vi "WS1050 16 DUT Reliability HD_Cycling Ver1.8.vi"() -> ()   [LabVIEW 2012]
uses:
  WS_VCAP Driver 024/Source/WSVCAP Shell/Type Defs/WSVCAP SHL I2C DUT Mask Mode Enum.ctl
  <vilib>/Utility/file.llb/Read From Spreadsheet File (DBL).vi
panel:
  out "VISA resource name out":refnum<visa-resource-name>="GPIB0::3::INSTR"
  out "error out 2":errorcluster={"status"=TRUE, "code"=-63192, "source"="niLvFpga_Open_PXI-7813R.vi"}
  in  "Reg1_Bit Cntrl":string[](array[string])=["01", "02", "04", "08", "10", "20", "40", "80", "03", "06", "0C", "D8", "33", "66", "CC", "07", "0E", "1C", "38", "70", "E0", "0F", "1E", "3C", "78", "F0", "1F", "3E", "7C", "F8", "3F", "7E", "FC", "7F", "FE", "FD", "FB", "F7", "EF", "DF", "BF", "7F", "FC", "F9", "F3", "E7", "CF", "9F", "3F", "F8", "F1", "E3", "C7", "8F", "1F", "F0", "E1", "C3", "87", "0F", "E0", "C1", "83", "07", "C0", "81", "03", "AA", "55", "00"]
  out "date string":string="5/19/2014"
  out "PS1 Out":refnum<visa-resource-name>
  out "Ke2000 Out":refnum<visa-resource-name>="GPIB0::9::INSTR"
  in  "Tab Control":T1(tab)
  in  "No of Cmd":i64=3
  in  "Serial Number":string[][](table)=[["DUT", "SN"], ["DUT1", "1"], ["DUT2", "2"], ["DUT3", "3"], ["DUT4", "4"], ["DUT5", "5"], ["DUT6", "6"], ["DUT7", "7"], ["DUT8", "8"], ["DUT9", "9"], ["DUT10", "10"], ["DUT11", "11"], ["DUT12", "12"], ["DUT13", "13"], ["DUT14", "14"], ["DUT15", "15"], ["DUT16", "16"]]
  out "AD7747 Values":string[][](table)
  in  "SPI Clock Rate (Hz)":dbl=5000000.0 caption="Cycle Speed" format="%.1p Hz"
  in  "Lot#":string="3T9BB"
  in  "Wafer#":string="25-EB"
  in  "File Name":string="CYC_3T9BB_25_EB_65C_40V_50DC_BRD3_141107_1"
  in  "TMN DC\\CAP Data Log File Path":path=path "C:/WS1050 16 DUT Data"
  in  "Test Program":string="WS1050 16 DUT Reliability HD_Cycling Ver1.8"
  out "Current Date":string="8/28/2014"
  out "Current Time":string="0950"
  in  "Start Date":string="4/24/2014"
  in  "Start Time":string="1542"
  in  "Comment":string="CYC65C40V"
  in  "OK Button":bool
  in  "Calibration":bool
  in  "Verify CP":bool
  in  "CP Setting":i32(ring) items=["CP OFF", "CP ON", "CP 35V", "CP 40V", "DVA ON", "DVA OFF", "REG1 ON", "REG1 OFF", "REG2 ON", "REG2 OFF", "REG3 ON", "REG3 OFF"]
  in  "Set VDD":dbl=3.7 format="%.3g"
  in  "Command":string[](array[string])=["0702013B3B3B", "0702013B3B3B", "070201000000"]
  in  "SPI Clock Rate (Hz)":dbl=1000000.0 caption="Meas Speed" format="%.1p Hz"
  out "AR  Meas(Hz)":dbl
  in  "PS1 Source":refnum<visa-resource-name>="GPIB0::5::INSTR"
  in  "Ke2000":refnum<visa-resource-name>="GPIB0::9::INSTR"
  in  "CP to HD/Cycle":i32(ring)=1 items=["CP HDC 35V", "CP HDC 40.25V", "CP HDC 27.5V", "CP HDC 30.5V", "CP HDC 44V"]
  out "Simulate FPGA":bool
  out "Online":bool
  out "AR Cycling(Hz)":dbl=5000000.0
  in  "Ke2400":refnum<visa-resource-name>="GPIB0::3::INSTR"
  in  "Initialize AD7747":bool
  in  "DUT Mask Mode":T2=enum."All"
  in  "RFFE Slave Address":u8=7 caption="Slave Address" format="0x%02x"
  out "Activity Log":string="05/19/2014 -- 12:24:35.853::WSVCAP::APP::Application Started\n05/19/2014 -- 12:24:37.606::WSVCAP::WSVCAP SHL::WR I2C-REG:0x0A;MASK:0xFFFFFFFFFFFF;C1 DATA:22:22:22:22:22:22:22:22:22:22:22:22:22:22:22:22;C2 DATA:22:22:22:22:22:22:22:22:22:22:22:22:22:22:22:22;C3 DATA:22:22:22:22:22:22:22:22:22:22:22:22:22:22:22:22\r\n05/19/2014 -- 12:24:37.773::WSVCAP::WSVCAP SHL::WR I2C-ST:0,0,4,1\r\n05/19/2014 -- 12:24:37.903::WSVCAP::WSVCAP SHL::RD I2C-BYTES:4;ADD:0x00;MASK:0xFFFFFFFFFFFF\r\n05/19/2014 -- 12:24:38.045::WSVCAP::WSVCAP SHL::RD I2C:C1 DATA:2:2:2:2:2:2:2:2:2:2:2:2:2:2:2:2|A7:A9:AA:82:82:7F:82:81:82:81:83:82:81:82:82:81|46:36:BB:88:44:A3:E9:2B:32:20:ED:25:BB:3D:68:B|2C:6A:EB:A7:22:56:FE:CC:36:82:D7:B0:3B:48:F9:CC;C2 DATA:2:2:2:2:2:2:2:2:2:2:2:2:2:2:2:2|94:94:94:80:80:80:80:80:81:7E:7E:81:80:7E:80:80|47:33:15:82:62:B:E8:1C:D7:C3:7D:41:7C:B7:4C:2A|C4:B4:AE:8:1E:D1:4E:37:11:C0:6F:63:42:9D:63:B5;C3 DATA:2:2:2:2:2:2:2:2:2:2:2:2:2:2:2:2|95:95:95:81:81:7E:81:80:84:7D:80:83:81:7E:7F:80|AB:C4:14:B5:7B:52:DF:C9:79:5D:5F:30:99:31:1E:F4|6E:5C:F7:A8:C3:EB:7B:EF:33:92:89:77:4D:67:75:DD;STATUS:0:0:4:0\r\n05/19/2014 -- 12:24:38.046::WSVCAP::WSVCAP SHL::WR I2C-REG:0x0A;MASK:0xFFFFFFFFFFFF;C1 DATA:22:22:22:22:22:22:22:22:22:22:22:22:22:22:22:22;C2 DATA:22:22:22:22:22:22:22:22:22:22:22:22:22:22:22:22;C3 DATA:22:22:22:22:22:22:22:22:22:22:22:22:22:22:22:22\r\n05/19/2014 -- 12:24:38.089::WSVCAP::WSVCAP SHL::WR I2C-ST:0,0,4,1\r\n05/19/2014 -- 12:24:38.219::WSVCAP::WSVCAP SHL::RD I2C-BYTES:4;ADD:0x00;MASK:0xFFFFFFFFFFFF\r\n05/19/2014 -- 12:24:38.362::WSVCAP::WSVCAP SHL::RD I2C:C1 DATA:2:2:2:2:2:2:2:2:2:2:2:2:2:2:2:2|A7:AB:AA:82:82:82:83:83:82:82:82:82:7F:82:82:81|4B:32:96:83:3E:61:43:17:25:62:AB:4D:A2:40:2E:5|3C:76:2B:B4:EE:E4:A9:1A:AA:A:26:C7:21:2E:87:5B;C2 DATA:2:2:2:2:2:2:2:2:2:2:2:2:2:2:2:2|94:94:94:80:80:80:80:80:80:7F:80:81:80:80:7F:80|4A:32:19:7D:19:6C:79:46:61:7F:4B:B8:A5:30:F3:14|B4:70:A:8C:9C:DC:43:FA:1E:A:C6:21:A:A9:13:F3;C3 DATA:2:2:2:2:2:2:2:2:2:2:2:2:2:2:2:2|95:97:94:81:80:81:82:81:80:7E:81:84:7F:81:80:80|B2:32:D0:A7:9E:4C:AB:D4:EE:D9:F0:82:B7:91:7:FF|C1:91:B6:3D:D8:E:1B:4F:9F:6A:F1:6C:E7:3F:7:BA;STATUS:0:0:4:0\r\n05/19/2014 -- 12:24:38.364::WSVCAP::WSVCAP SHL::WR I2C-REG:0x0A;MASK:0xFFFFFFFFFFFF;C1 DATA:22:22:22:22:22:22:22:22:22:22:22:22:22:22:22:22;C2 DATA:22:22:22:22:22:22:22:22:22:22:22:22:22:22:22:22;C3 DATA:22:22:22:22:22:22:22:22:22:22:22:22:22:22:22:22\r\n05/19/2014 -- 12:24:38.406::WSVCAP::WSVCAP SHL::WR I2C-ST:0,0,4,1\r\n05/19/2014 -- 12:24:38.536::WSVCAP::WSVCAP SHL::RD I2C-BYTES:4;ADD:0x00;MASK:0xFFFFFFFFFFFF\r\n05/19/2014 -- 12:24:38.678::WSVCAP::WSVCAP SHL::RD I2C:C1 DATA:2:2:2:2:2:2:2:2:2:2:2:2:2:2:2:2|A7:A9:AB:82:82:81:82:82:82:82:82:82:82:82:82:81|46:71:4C:87:43:3D:7F:FC:25:4F:8E:54:97:3E:60:8C|AA:F4:1F:B5:CE:43:1F:36:9:87:9C:78:86:5:B6:8E;C2 DATA:2:2:2:2:2:2:2:2:2:2:2:2:2:2:2:2|94:94:94:80:7F:7F:80:80:80:80:80:81:80:80:80:80|49:36:18:7D:6E:C5:E4:3C:81:2E:41:D3:75:71:E3:72|E8:D3:E6:D1:E0:48:AE:D4:54:D:E8:8E:B4:41:68:4;C3 DATA:2:2:2:2:2:2:2:2:2:2:2:2:2:2:2:2|95:95:95:81:7F:7F:81:81:81:81:81:84:81:81:82:81|B3:F5:90:AB:82:69:7B:93:D0:77:E8:D5:E8:8C:84:E8|B9:AC:EE:2B:B6:71:8F:4A:74:31:56:BB:8A:B7:A0:C8;STATUS:0:0:4:0\r\n05/19/2014 -- 12:24:38.681::WSVCAP::WSVCAP SHL::WR I2C-REG:0x0A;MASK:0xFFFFFFFFFFFF;C1 DATA:22:22:22:22:22:22:22:22:22:22:22:22:22:22:22:22;C2 DATA:22:22:22:22:22:22:22:22:22:22:22:22:22:22:22:22;C3 DATA:22:22:22:22:22:22:22:22:22:22:22:22:22:22:22:22\r\n05/19/2014 -- 12:24:38.723::WSVCAP::WSVCAP SHL::WR I2C-ST:0,0,4,1\r\n05/19/2014 -- 12:24:38.854::WSVCAP::WSVCAP SHL::RD I2C-BYTES:4;ADD:0x00;MASK:0xFFFFFFFFFFFF\r\n05/19/2014 -- 12:24:38.996::WSVCAP::WSVCAP SHL::RD I2C:C1 DATA:2:2:2:2:2:2:2:2:2:2:2:2:2:2:2:2|A7:A9:AA:82:82:7F:83:81:82:81:84:82:7F:82:7F:82|43:FB:E:7F:3C:AD:35:35:26:A2:6C:21:4B:3D:8:6|63:9A:E1:F3:95:32:91:42:90:3C:78:1F:5C:D7:5F:D8;C2 DATA:2:2:2:2:2:2:2:2:2:2:2:2:2:2:2:2|94:94:94:80:80:80:80:80:81:80:7E:81:80:7E:7F:80|48:36:18:7F:5E:3D:69:83:DE:AE:A1:9E:31:AE:BB:96|15:A0:44:17:13:FD:CC:C8:6D:B2:EF:A7:C:C7:3B:F;C3 DATA:2:2:2:2:2:2:2:2:2:2:2:2:2:2:2:2|95:96:94:81:81:7E:82:80:84:80:80:84:7F:7E:7D:82|AD:3B:6D:A9:7C:57:9D:F5:7A:96:23:5C:36:2D:ED:5A|CD:46:DB:3B:C7:BD:70:60:33:B8:B:F7:63:A:51:4D;STATUS:0:0:4:0\r\n05/19/2014 -- 12:24:38.998::WSVCAP::WSVCAP SHL::WR I2C-REG:0x0A;MASK:0xFFFFFFFFFFFF;C1 DATA:22:22:22:22:22:22:22:22:22:22:22:22:22:22:22:22;C2 DATA:22:22:22:22:22:22:22:22:22:22:22:22:22:22:22:22;C3 DATA:22:22:22:22:22:22:22:22:22:22:22:22:22:22:22:22\r\n05/19/2014 -- 12:24:39.040::WSVCAP::WSVCAP SHL::WR I2C-ST:0,0,4,1\r\n05/19/2014 -- 12:24:39.170::WSVCAP::WSVCAP SHL::RD I2C-BYTES:4;ADD:0x00;MASK:0xFFFFFFFFFFFF\r\n05/19/2014 -- 12:24:39.311::WSVCAP::WSVCAP SHL::RD I2C:C1 DATA:2:2:2:2:2:2:2:2:2:2:2:2:2:2:2:2|A7:AA:AB:82:82:81:82:81:82:81:82:82:82:82:7F:82|44:F1:90:87:45:44:C8:2C:2C:F1:FC:1B:94:3B:3C:75|4A:49:95:19:99:73:64:3:23:24:F3:A2:5E:7F:C4:B6;C2 DATA:2:2:2:2:2:2:2:2:2:2:2:2:2:2:2:2|94:94:94:80:80:80:80:7F:80:80:7E:80:80:7E:7F:80|4C:36:17:7D:A8:9F:DE:C7:53:6D:8A:F4:41:A5:C6:E0|90:2E:24:C:D9:22:E4:76:3B:40:1D:53:33:B1:3E:4D;C3 DATA:2:2:2:2:2:2:2:2:2:2:2:2:2:2:2:2|95:97:95:81:81:7F:81:80:80:81:7F:82:81:7E:7D:82|AE:2B:A7:AB:CC:CD:A4:38:FD:17:80:F2:92:2D:45:C4|76:E5:D:B9:AD:B5:BA:8D:28:32:9E:42:B7:20:4A:D9;STATUS:0:0:4:0\r\n05/19/2014 -- 12:24:39.313::WSVCAP::WSVCAP SHL::WR I2C-REG:0x0A;MASK:0xFFFFFFFFFFFF;C1 DATA:22:22:22:22:22:22:22:22:22:22:22:22:22:22:22:22;C2 DATA:22:22:22:22:22:22:22:22:22:22:22:22:22:22:22:22;C3 DATA:22:22:22:22:22:22:22:22:22:22:22:22:22:22:22:22\r\n05/19/2014 -- 12:24:39.355::WSVCAP::WSVCAP SHL::WR I2C-ST:0,0,4,1\r\n05/19/2014 -- 12:24:39.486::WSVCAP::WSVCAP SHL::RD I2C-BYTES:4;ADD:0x00;MASK:0xFFFFFFFFFFFF\r\n05/19/2014 -- 12:24:39.628::WSVCAP::WSVCAP SHL::RD I2C:C1 DATA:2:2:2:2:2:2:2:2:2:2:2:2:2:2:2:2|A7:A9:AA:82:82:82:83:82:82:82:82:82:7F:82:7F:82|47:18:E4:87:3E:E7:6:65:25:92:37:38:A8:3E:89:85|7C:A7:7:2B:A3:7A:EC:EF:89:ED:F4:D3:D8:BC:3A:F5;C2 DATA:2:2:2:2:2:2:2:2:2:2:2:2:2:2:2:2|94:94:94:80:7F:80:80:7F:81:80:7E:80:80:80:81:80|49:37:17:80:76:25:6A:F8:DF:55:97:4D:B8:5B:2B:B1|13:E3:9A:3E:1A:2D:4F:B6:DB:E9:61:FA:8B:D6:9:CC;C3 DATA:2:2:2:2:2:2:2:2:2:2:2:2:2:2:2:2|95:95:95:81:7F:80:82:81:84:80:7F:81:80:81:7F:82|AF:93:3B:AF:5B:11:82:E4:7E:C3:2D:72:9:96:D9:A|DB:96:F2:10:5F:64:9A:C6:98:12:27:7D:10:D3:20:D9;STATUS:0:0:4:0\r\n05/19/2014 -- 12:24:40.132::WSVCAP::WSVCAP SHL::CLOSE\r\n"
  in  "C1 Cap DAC":u8=128 caption="B Data In" format="0x%02x"
  in  "C2 Cap DAC":u8=128 caption="B Data In" format="0x%02x"
  in  "C3 Cap DAC":u8=128 caption="B Data In" format="0x%02x"
  out "IDD Brd(uA)":string
  in  "CP to Meas":i32(ring)=1 items=["CP HDC 35V", "CP HDC 40.25V", "CP HDC 27.5V", "CP HDC 30.5V", "CP HDC 44V"]
  in  "Set Delay":dbl[](array[numeric])=[1.8e-05, 1.8e-05, 1.8e-05] min=0.0 max=0.5 format="%#.0p s"
  in  "CP VPI":i32(ring) items=["CP HDC 35V", "CP HDC 40.25V", "CP HDC 27.5V", "CP HDC 30.5V", "CP HDC 44V"]
  in  "Real No. From\nLookup Table":bool
  in  "Control Panel":T3={"Verify Socket"=FALSE, "HD/CYC"=FALSE, "E-CAL"=FALSE, "DVA"=FALSE, "VPI"=TRUE, "VSA"=TRUE, "HS"=TRUE}
  out "Verify Socket":bool
  out "HD/CYC":bool
  out "E-CAL":bool
  out "DVA":bool
  out "VPI":bool
  out "VSA":bool
  out "HS":bool
  in  "Repeat Meas(s)":u32=300
  in  "Freq(Hz)":string="12K"
  in  "Brd #":string="1"
  out "error out":errorcluster
  in  "error in (no error)":errorcluster
  in  "WS1050/51":bool=TRUE
  in  "Test Sequences":i32(ring) items=["C1_C2_C3", "C2_C1_C3", "C3_C2_C1"]
  in  "%Duty Cycle":string="33"
  in  "Cmin/Act":bool
  in  "Cmd to HD":string="070201383838"
  out "40V_1":string[][](table)
  out "VPI C1":string[][](table)
  out "VPI C3":string[][](table)
  out "NOM IDD OFF(uA)":string
  out "40V_2":string[][](table)
  out "VPI C2":string[][](table)
  out "NOM IDD ON (uA)":string
  out "40V_3":string[][](table)
  out "Total Time":u64
  out "IDD Stdby(uA)":string="2.606990E+0"
  out "EFuse RB T0":string[](array[string])
  out "Current EFuse Read back":string[](array[string])
  in  "Set HD/Cycle \nto Complete":u64=50000000000
  out "No of HD/Cycle\nCompleted":u64
  out "Cycle Count":u64 min=1 max=4 step=1
  out "Loop \ncompleted":i32=1
  out "Previous Time":string="12:20:26 PM"
  out "STATUS":string="Idle...."
  out "IDD_HD/CYC (uA)":string="164.601255E+0"
  in  "stop During HD/Cycles":bool
  in  "stop":bool
  out "Total Delta 2(pF)":string[](array[string])
  out "Total Delta 1(pF)":string[](array[string])
  out "Total Delta 3(pF)":string[](array[string])
  out "% Delta C_T0":string[][](array[string])
  out "% Delta C":string[][](array[string])
  out "EFuse Readback Status":bool[](array[boolean])
  in  "DeltaC Target(pF)_50":dbl=7.375
  out "RB Reg for HD":string[](array[string])
  out "RB Reg for HD/Cycle":string[](array[string])
  in  "DeltaC Target(pF)_51":dbl=5.875
  out "VSA_V1":string[][](table)
  out "VSA_V2":string[][](table)
  out "VSA_V3":string[][](table)
  in  "VSA Voltage(V)":dbl[](array[numeric])=[-10.0, 0.0, 10.0]
  in  "DC_Temp":i32=65
  in  "HD/CYC Temp":i32=65
  in  "Time All ON (s)":u32=120
  in  "Time All OFF (s)":u32=120
  in  "HD_DC (Min)":u64=259200
  out "LPs Count":i32
  in  "X Repeat":i32=100
  out "No LPs to RP":i32
  out "Running Loops":i32=1
  out "TTime Completed":u64=2000
  in  "TTF Completed":u64=50000000000
  in  "HD RP(Min)":dbl=60.0
  in  "CYC RP (X1000)":dbl=10000.0
  out "Min Plot_1":dbl[][](graph) caption="(Y) Multi Plot 2"
  out "Min Plot_2":dbl[][](graph) caption="(Y) Multi Plot 2"
  out "Min Plot_3":dbl[][](graph) caption="(Y) Multi Plot 2"
  in  "Debug":bool
  in  "No of Rows\nFrom Spread Sheet":i32
  in  "Plot Delta Cmin":bool=TRUE
  in  "Plot":T4(ring)
  # "Company:  WiSpry Inc\n20 Fairbanks Ste 198 Irvine CA 92618\n\nAuthor:  Andy V Tran\nCreated:  09/14/2015\nLabVIEW 2012 Pro\nTP:  WS1050 16 DUT HD/Cycle ver1.8\nFPGA Version: WS_VCAP Driver 024"
  # "Note for HD during Cycles Setup:\n\n1.  Set HD/Cycle to Completed = 4320 minutes = 72 hours \n(T0 24hrs HD, T2 48hrs HD_Duty Cycle);  Default Setting\n2.  Set Time to Start HD Duty Cycle = 1440 = 24 hours\n3.  Set Time All ON = 120s = 2 minutes\n4.  Set Time All OFF = 120s = 2 minutes\n5.  No of Loops to RP = 3600s/(Time ALL ON(s) + Time ALL + OFF(s))\n6.  X Repeat = X runs\n7.  Set TTF Completed = Repeat X item1 to Stop.\n8.  Stop Test, set TTF Completed = Total Time Completed.\n\nNote for Cycling:\n\n\n\nVersion 1.8 is the latest verision for WS1050 16 DUT test program.\n\n1.  Added Stress Sequences,\n2.  Added CMin/ON-OFF Repeat Measurement\n3.  Fill \"na\" when no test"
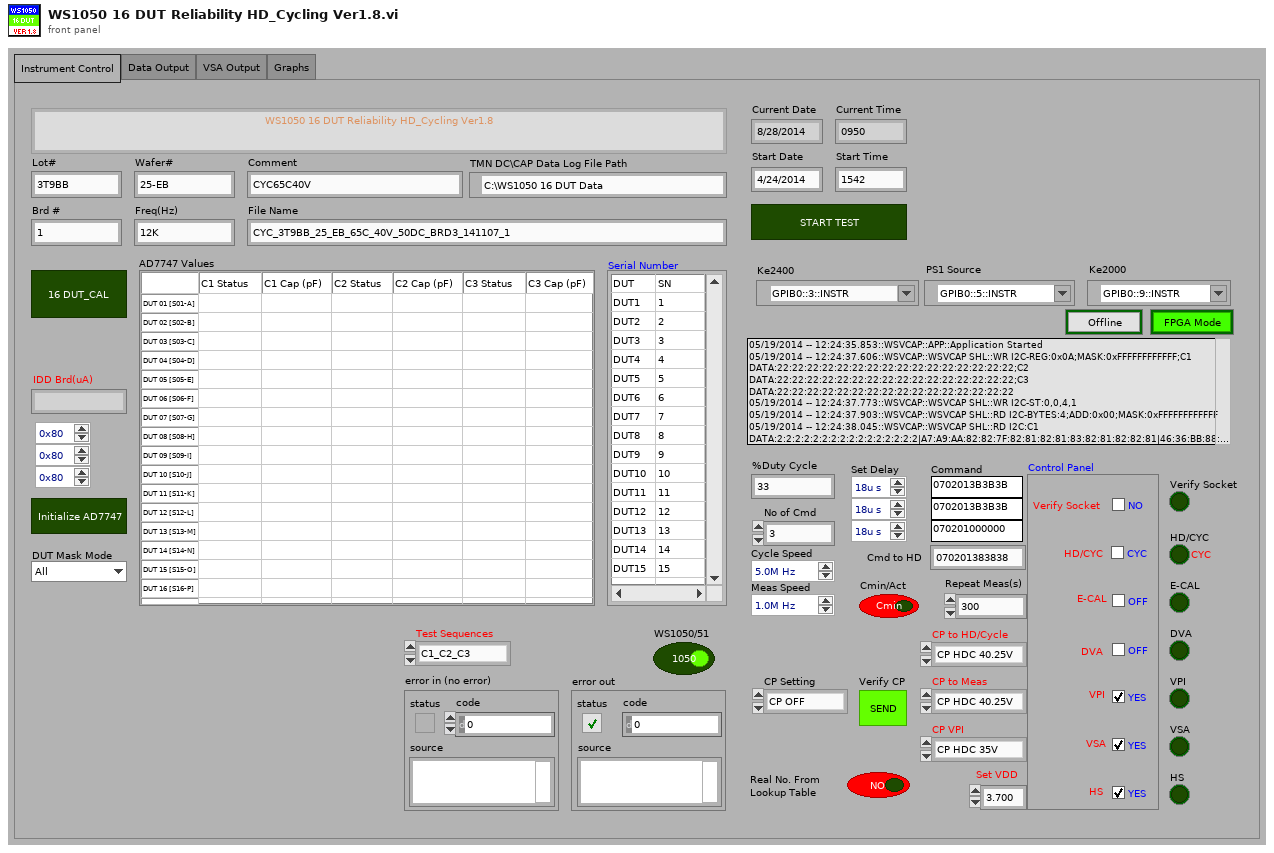
[diagram p1: front panel]
types:
  T1 = enum32{"Instrument Control", "Data Output", "VSA Output", "Graphs"}
  T2 = typedef "WSVCAP SHL I2C DUT Mask Mode Enum.ctl" = enum16{"Custom", "C1", "C2", "C3", "All"}
  T3 = cluster{"Verify Socket":bool, "HD/CYC":bool, "E-CAL":bool, "DVA":bool, "VPI":bool, "VSA":bool, "HS":bool}
  T4 = enum16{"DUT ALL", "DUT 01", "DUT 02", "DUT 03", "DUT 04", "DUT 05", "DUT 06", "DUT 07", "DUT 08", "DUT 09", "DUT 10", "DUT 11", "DUT 12", "DUT 13", "DUT 14", "DUT 15", "DUT 16"}
  T5 = typedef "WSVCAP SHL Core System Cluster.ctl" = cluster{"Settings":T6, "FPGA Resource":tag, "Online":bool, "I2C Wait Ticks":u32, "SPI Wait Ticks":u32, "RFFE Wait Ticks":u32}
  T6 = typedef "WSVCAP SHL I2C Settings Cluster.ctl" = cluster{"FPGA Resource Name":string, "I2C Slave Address":u8, "I2C Clock Rate (Hz)":dbl, "SPI Clock Rate (Hz)":dbl, "RFFE Slave Address":u8, "RFFE Clock Rate (Hz)":dbl, "Simulate FPGA":bool, "C1 Cap DAC Default":u8, "C2 Cap DAC Default":u8, "C3 Cap DAC Default":u8}
  T7 = enum16{"Idle...", "Voltage 1", "Voltage 2", "Voltage 3"}[]
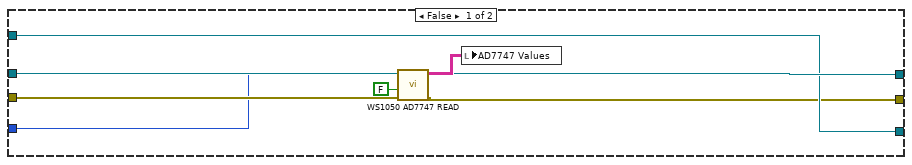
[diagram p9: hidden frame]
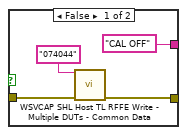
[diagram p10: hidden frame]
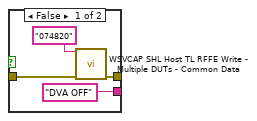
[diagram p11: hidden frame]
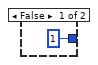
[diagram p12: hidden frame]
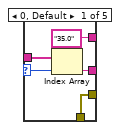
[diagram p13: hidden frame]
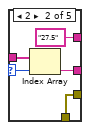
[diagram p14: hidden frame]
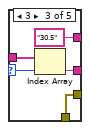
[diagram p15: hidden frame]
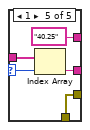
[diagram p16: hidden frame]
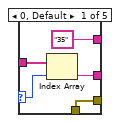
[diagram p17: hidden frame]
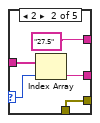
[diagram p18: hidden frame]
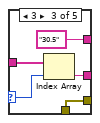
[diagram p19: hidden frame]
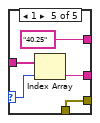
[diagram p20: hidden frame]
diagram:
  w7 = u16 0 items=["Off", "Moving Filter", "Repeating Filter"] ("Digital Filter (0: Off)")
  w12 = u16 7 items=["3.5 Digits"=4, "4.5 Digits"=5, "5.5 Digits"=6, "6.5 Digits"=7] ("Resolution (7: 6.5 digits)")
  w27 = TRUE
  n1 = case shown="True" w27 {
    tunnel: "error in (no error)" -> [w32 w33]
    tunnel: [w32 w40] -> w3
    frame False {
    }
    frame True {
      n2 = call "WSVCAP SHL Host TL Initialize.vi"("error in"=w33) -> ("error out"=w34:errorcluster)  [unwired: 13 in, 1 out]
      n3 = control-ref of="Activity Log"() -> (w36:refnum<vi>)
      n4 = call "ACT LG Activity Log Core.vi"("Display Ref"=w36, "Source"="WSVCAP", "Error In (no error)"=w34) -> ("Error Out"=w35:errorcluster)  [unwired: 11 in, 1 out]
      n5 = call "WSVCAP SHL Host TL Status Manager.vi"("error in"=w35) -> ("System Out"=w41:T5, "error out"=w40:errorcluster)  [unwired: 13 in]
      n6 = Unbundle By Name(w41) -> ("Online"=→"Online":bool, "Settings.Simulate FPGA"=→"Simulate FPGA":bool)
    }
  }
  n7 = case shown="True" TRUE {
    tunnel: w3 -> [w42 w47]
    tunnel: [w43 w46] -> w25
    tunnel: [w42 w45] -> w18
    tunnel: "Ke2400" -> [w43 w44]
    frame False {
    }
    frame True {
      n8 = VISA Write(VISA resource name=w44, write buffer="SOUR:FUNC VOLT;VOLT:MODE FIX;RANG 100;LEV 0.0;:SENS:FUNC \"CURR\";CURR:PROT 60E-3;RANG 100E-3;:OUTP ON", error in (no error)=w47) -> (VISA resource name out=w46:refnum<visa-resource-name>, error out=w45:errorcluster)  [unwired: 1 out]
    }
  }
  n9 = call "Ke2000 Configure DC Current.vi"("Resolution (7: 6.5 digits)"=w12, "Digital Filter (0: Off)"=w7, "Auto Range? (T: Auto)"=FALSE, "error in"=w3, "Custom Range (0 A)"=1.0, "VISA resource name"="Ke2000") -> ("error out"=w10:errorcluster, "VISA resource name out"=w9:refnum<visa-resource-name>)  [unwired: 4 in]
  n10 = call "Agilent 3631A Initialize.vi"("error in (no error)"=w3, "Default"=FALSE ("Reset? (T: Yes)"), "Reset"=TRUE ("ID Query? (T: Yes)"), "VISA resource name"="PS1 Source") -> ("error out"=w2:errorcluster, "VISA resource name out"=w1:refnum<visa-resource-name>)  [unwired: 6 in]
  n11 = case shown="True" TRUE {
    tunnel: [_ w49] -> w31
    frame False {
    }
    frame True {
      n12 = call-poly <vilib>:"Read From Spreadsheet File.vi"("number of rows (all:-1)"=-1) -> ("all rows"=w49:dbl[][])  [unwired: 6 in, 4 out]
    }
  }
  n13 = Merge Errors(w18, w10, w2) -> (w26:errorcluster)
  n14 = while {
    tunnel: w26 -> [w74]
    tunnel: [w62] -> w22
    tunnel: w31 -> [w79]
    tunnel: w1 -> [w66]
    tunnel: w9 -> [w67]
    tunnel: [w77] -> w30
    tunnel: [w76] -> w29
    tunnel: w25 -> [w73]
    tunnel: [w72] -> w23
    tunnel: [FALSE ("stop")] -> w16
    i -> [w75]
    stop <- w80 stop-if-true
    n15 = case shown="0" w75 {
      tunnel: w74 -> [w90 w92]
      tunnel: [w89 w92] -> w69
      tunnel: "RFFE Slave Address" -> [w87 _]
      frame 0 {
        w83 = dbl[][] []
        w82 = "" ("uA")
        w84 = string[][] []
        w85 = string[] [] ("EFuse Read back")
        w91 = u64 0 ("No of HD/Cycle\nCompleted")
        n16 = local write "RB Reg for HD/Cycle"(w85) -> ()
        n17 = local write "Current EFuse Read back"(w85) -> ()
        n18 = local write "EFuse RB T0"(w85) -> ()
        n19 = local write "No of HD/Cycle\nCompleted"(w91) -> ()
        n20 = local write "Cycle Count"(w91) -> ()
        n21 = local write "Total Delta 1(pF)"(w85) -> ()
        n22 = local write "Total Delta 2(pF)"(w85) -> ()
        n23 = local write "Total Delta 3(pF)"(w85) -> ()
        n24 = local write "VPI C2"(w84) -> ()
        n25 = local write "VSA_V3"(w84) -> ()
        n26 = local write "VSA_V1"(w84) -> ()
        n27 = local write "VSA_V2"(w84) -> ()
        n28 = local write "VPI C1"(w84) -> ()
        n29 = local write "VPI C3"(w84) -> ()
        n30 = local write "% Delta C"(w84) -> ()
        n31 = local write "% Delta C_T0"(w84) -> ()
        n32 = local write "40V_2"(w84) -> ()
        n33 = local write "40V_1"(w84) -> ()
        n34 = local write "40V_3"(w84) -> ()
        n35 = local write "NOM IDD OFF(uA)"(w82) -> ()
        n36 = local write "NOM IDD ON (uA)"(w82) -> ()
        n37 = local write "IDD Brd(uA)"(w82) -> ()
        n38 = local write "Min Plot_3"(w83) -> ()
        n39 = local write "Min Plot_1"(w83) -> ()
        n40 = local write "Min Plot_2"(w83) -> ()
        n41 = call "WSVCAP SHL Host TL RFFE Configure.vi"("RFFE Slave Address"=w87, "Clock Rate (Hz)"="SPI Clock Rate (Hz)", "error in"=w90) -> ("Actual Rate (Hz)"=→"AR  Meas(Hz)":dbl, "error out"=w89:errorcluster)  [unwired: 11 in]
      }
      frame 1, Default {
      }
    }
    n42 = while {
      tunnel: ["stop"] -> w71
      tunnel: w69 -> [w117]
      tunnel: [w108] -> w63
      tunnel: w66 -> [w115]
      tunnel: w67 -> [w110]
      tunnel: [w111] -> w65
      tunnel: [w109] -> w64
      tunnel: [w104] -> w61
      tunnel: [w103] -> w60
      tunnel: [w102] -> w59
      tunnel: [w101] -> w58
      tunnel: [w100] -> w57
      tunnel: [w99] -> w56
      tunnel: [w98] -> w55
      tunnel: ["Command"] -> w54
      tunnel: ["Set Delay"] -> w53
      stop <- w124 stop-if-true
      # "Set Date & Time to Start Test"
      n43 = case shown="True" "Initialize AD7747" {
        tunnel: w117 -> [w133 w138]
        tunnel: [w133 w134] -> w116
        tunnel: w115 -> [w132 w136]
        tunnel: [w132 w135] -> w114
        frame False {
        }
        frame True {
          w139 = T7 [enum."Voltage 2", enum."Voltage 3", enum."Voltage 1"] items=["Idle...", "Voltage 1", "Voltage 2", "Voltage 3"]
          n44 = for {
            tunnel: w136 -> [w149]
            tunnel: w139 -> [w146] mode=indexing
            tunnel: [w145] -> w135
            shift-right: [w141] -> w137
            shift-left: w138 -> [w150]
            n45 = local read "Set VDD"() -> (w144:dbl)
            n46 = call "E3631A_Voltage Controller updated.vi"("VISA resource name"=w149, "I_VDD(A)"=0.2, "Channel Controller"=w146, "Voltage 1"=w144, "Voltage 2"=3.3, "error in (no error)"=w150, "Voltage 3"=-3.3) -> ("VISA resource name out"=w145:refnum<visa-resource-name>, "error out"=w140:errorcluster)  [unwired: 7 in]
            n47 = call "Delay T4.vi"("milliseconds to wait"=u32 100, "error in (no error)"=w140) -> ("error out"=w141:errorcluster)  [unwired: 9 in]
          }
          n48 = call "WS1050_AD7747_Init.vi"("error in"=w137) -> ("error out"=w134:errorcluster)  [unwired: 10 in]
        }
      }
      n49 = call "Time_stamp.vi"() -> ("date/time string"=w129:string, "date string"=w131:string)  [unwired: 2 in]
      "Current Date" <- w131
      "Current Time" <- w129
      n50 = Equal?(x=w131, y="Start Date") -> (x = y?=w127:bool)
      n51 = Equal?(x=w129, y="Start Time") -> (x = y?=w126:bool)
      n52 = And(x=w127, y=w126) -> (x .and. y?=w123:bool)
      n53 = Compound Arithmetic op=OR(w123, "OK Button", "stop") -> (w124:bool)
      n54 = case shown="True" "Calibration" {
        tunnel: w116 -> [w179 w197]
        tunnel: [w174 w194] -> w106
        tunnel: w114 -> [w178 w193]
        tunnel: "DUT Mask Mode" -> [w177 w189]
        tunnel: [w178 w188] -> w112
        tunnel: w110 -> [w176 w184]
        tunnel: [w176 w181] -> w109
        frame False {
          n55 = call "WS1050 AD7747 READ.vi"("error in"=w179, "Log (T)"=FALSE, "DUT Mask Mode (All)"=w177) -> ("error out"=w174:errorcluster, "AD7747 Values"=w180:string[][])  [unwired: 7 in]
          n56 = local write "AD7747 Values"(w180) -> ()
        }
        frame True {
          n57 = flat-sequence {
            tunnel: w197 -> [w206]
            tunnel: [w201] -> w196
            tunnel: w193 -> [w205]
            tunnel: [w204] -> w192
            tunnel: w189 -> [w203]
            tunnel: [w203] -> w190
            tunnel: w184 -> [w199]
            tunnel: [w198] -> w183
            tunnel: w196 -> [w234]
            tunnel: [w221] -> w195
            tunnel: w192 -> [w233]
            tunnel: [w233] -> w191
            tunnel: w190 -> [w232]
            tunnel: "C1 Cap DAC" -> [w228]
            tunnel: "C2 Cap DAC" -> [w227]
            tunnel: "C3 Cap DAC" -> [w226]
            tunnel: w183 -> [w225]
            tunnel: [w225] -> w182
            tunnel: w195 -> [w237]
            tunnel: [w240] -> w194
            tunnel: w191 -> [w239]
            tunnel: [w236] -> w188
            tunnel: w182 -> [w235]
            tunnel: [w235] -> w181
            frame #0 {
              w207 = T7 [enum."Voltage 2", enum."Voltage 3", enum."Voltage 1"] items=["Idle...", "Voltage 1", "Voltage 2", "Voltage 3"]
              n58 = for {
                tunnel: w205 -> [w218]
                tunnel: w207 -> [w215] mode=indexing
                tunnel: [w214] -> w204
                shift-right: [w212] -> w200
                shift-left: w206 -> [w219]
                n59 = local read "Set VDD"() -> (w209:dbl)
                n60 = call "E3631A_Voltage Controller updated.vi"("VISA resource name"=w218, "I_VDD(A)"=0.2, "Channel Controller"=w215, "Voltage 1"=w209, "Voltage 2"=3.3, "error in (no error)"=w219, "Voltage 3"=-3.3) -> ("VISA resource name out"=w214:refnum<visa-resource-name>, "error out"=w211:errorcluster)  [unwired: 7 in]
                n61 = call "Delay T4.vi"("milliseconds to wait"=u32 100, "error in (no error)"=w211) -> ("error out"=w212:errorcluster)  [unwired: 9 in]
              }
              n62 = call "Ke2000 Single Reading.vi"("error in (no error)"=w200, "VISA resource name"=w199) -> ("error out"=w201:errorcluster, "VISA resource name out"=w198:refnum<visa-resource-name>, "uA"=→"IDD Brd(uA)":string)  [unwired: 5 in, 2 out]
              n63 = One Button Dialog(message="Please verify all sockets should be empty...") -> ()  [unwired: 1 in, 1 out]
            }
            frame #1 {
              # "Calibration Multi-Sockets"
              n64 = call "WS1050 CAPDAC Setting.vi"("DUT Mask Mode (All)"=w232, "error in"=w234, "C3 Cap DAC"=w226, "C2 Cap DAC"=w227, "C1 Cap DAC"=w228) -> ("error out"=w230:errorcluster)  [unwired: 5 in, 1 out]
              n65 = call "WS1050 OFFSET CAL.vi"("error in"=w230, "OFFSET CAL"=TRUE ("Read?")) -> ("error out"=w229:errorcluster)  [unwired: 8 in, 1 out]
              n66 = call "WS1050 AD7747 READ.vi"("error in"=w229, "Log (T)"=FALSE, "DUT Mask Mode (All)"=w232) -> ("error out"=w222:errorcluster, "AD7747 Values"=→"AD7747 Values":string[][])  [unwired: 7 in]
              n67 = call "Delay T4.vi"("milliseconds to wait"=u32 50, "error in (no error)"=w222) -> ("error out"=w221:errorcluster)  [unwired: 9 in]
            }
            frame #2 {
              w238 = T7 [enum."Voltage 2", enum."Voltage 3", enum."Voltage 1"] items=["Idle...", "Voltage 1", "Voltage 2", "Voltage 3"]
              n68 = for {
                tunnel: w239 -> [w252]
                tunnel: w238 -> [w248] mode=indexing
                tunnel: [w247] -> w236
                shift-right: [w243] -> w240
                shift-left: w237 -> [w249]
                n69 = call "E3631A_Voltage Controller updated.vi"("VISA resource name"=w252, "I_VDD(A)"=0.2, "Channel Controller"=w248, "Voltage 1"=0.0, "Voltage 2"=3.3, "error in (no error)"=w249, "Voltage 3"=-3.3) -> ("VISA resource name out"=w247:refnum<visa-resource-name>, "error out"=w242:errorcluster)  [unwired: 7 in]
                n70 = call "Delay T4.vi"("milliseconds to wait"=u32 100, "error in (no error)"=w242) -> ("error out"=w243:errorcluster)  [unwired: 9 in]
              }
              n71 = One Button Dialog(message="Calibration Completed....") -> ()  [unwired: 1 in, 1 out]
            }
          }
        }
      }
      n72 = call "Control Panel.vi"("error in (no error)"=w106, "Control Panel"="Control Panel") -> ("error out"=w105:errorcluster, "VPI"=w100:bool, "DVA"=w101:bool, "E-CAL"=w102:bool, "VSA"=w99:bool, "HD/CYC"=w103:bool, "HS"=w98:bool, "Verify Socket"=w104:bool)  [unwired: 2 in]
      "Verify Socket" <- w104
      "HS" <- w98
      "VSA" <- w99
      "VPI" <- w100
      "E-CAL" <- w102
      "HD/CYC" <- w103
      "DVA" <- w101
      n73 = case shown="True" "Verify CP" {
        tunnel: [w151 w154] -> w108
        tunnel: w112 -> [w152 w159]
        tunnel: [w152 w157] -> w111
        tunnel: w105 -> [w151 w156]
        frame False {
        }
        frame True {
          w160 = T7 [enum."Voltage 2", enum."Voltage 3", enum."Voltage 1"] items=["Idle...", "Voltage 1", "Voltage 2", "Voltage 3"]
          # "Verify CP"
          n74 = for {
            tunnel: w159 -> [w172]
            tunnel: w160 -> [w169] mode=indexing
            shift-right: [w166] -> w158
            shift-left: w156 -> [w173]
            tunnel: [w164] -> w157
            n75 = local read "Set VDD"() -> (w168:dbl)
            n76 = call "E3631A_Voltage Controller updated.vi"("VISA resource name"=w172, "Channel Controller"=w169, "Voltage 1"=w168, "Voltage 2"=3.3, "error in (no error)"=w173, "Voltage 3"=-3.3) -> ("VISA resource name out"=w164:refnum<visa-resource-name>, "error out"=w167:errorcluster)  [unwired: 8 in]
            n77 = call "Delay T4.vi"("milliseconds to wait"=u32 100, "error in (no error)"=w167) -> ("error out"=w166:errorcluster)  [unwired: 9 in]
          }
          n78 = Index Array(array=string[] ["074000", "074040", "07476F", "074776", "074800", "074820", "07413B", "074100", "07423B", "074200", "07433B", "074300"], index="CP Setting") -> (element=w161:string)
          n79 = call "WSVCAP SHL Host TL RFFE Write - Multiple DUTs - Common Data.vi"("Data Out"=w161, "error in"=w158) -> ("error out"=w155:errorcluster)  [unwired: 13 in]
          n80 = call "Delay T4.vi"("milliseconds to wait"=u32 10, "error in (no error)"=w155) -> ("error out"=w154:errorcluster)  [unwired: 9 in]
        }
      }
      n81 = Array Subset(array="Set Delay", length="No of Cmd") -> (w95:dbl[])  [unwired: 1 in]
      n82 = Array Subset(array="Command", length="No of Cmd") -> (w96:string[])  [unwired: 1 in]
      n83 = property on="Command" class="Arr (strict)"("Number of Rows"="No of Cmd") -> ()  [unwired: 2 in, 2 out]
      n84 = property on="Set Delay" class="Arr (strict)"("Number of Rows"="No of Cmd") -> ()  [unwired: 2 in, 2 out]
      n85 = local write "Command"(w96) -> ()
      n86 = local write "Set Delay"(w95) -> ()
      n87 = Wait Until Next ms Multiple(millisecond multiple=u32 100) -> ()  [unwired: 1 out]
    }
    n88 = case shown="False" w71 {
      tunnel: w63 -> [w310 w1840]
      tunnel: [w294 w1840] -> w62
      tunnel: w79 -> [w311 _]
      tunnel: w65 -> [w309 w1838]
      tunnel: w64 -> [w300 w1839]
      tunnel: [w307 w1839] -> w77
      tunnel: [w304 w1838] -> w76
      tunnel: w73 -> [w297 w1837]
      tunnel: [w293 w1837] -> w72
      tunnel: "RFFE Slave Address" -> [w288 _]
      tunnel: [w253 FALSE ("stop During HD/Cycles")] -> w51
      tunnel: w61 -> [w262 _]
      tunnel: w60 -> [w261 _]
      tunnel: w59 -> [w260 _]
      tunnel: w58 -> [w259 _]
      tunnel: w57 -> [w258 _]
      tunnel: w56 -> [w257 _]
      tunnel: w55 -> [w256 _]
      tunnel: w54 -> [w255 _]
      tunnel: w53 -> [w254 _]
      frame False {
        w289 = u64 0 ("Total Completed")
        w268 = u32 100 ("milliseconds to wait")
        w306 = T7 [enum."Voltage 2", enum."Voltage 3", enum."Voltage 1"] items=["Idle...", "Voltage 1", "Voltage 2", "Voltage 3"]
        w308 = T7 [enum."Voltage 2", enum."Voltage 3", enum."Voltage 1"] items=["Idle...", "Voltage 1", "Voltage 2", "Voltage 3"]
        # "DVA"
        # "Verify Socket"
        # "E-CAL"
        # "VSA"
        # "VPI"
        # "HS"
        # "DVA"
        # "HD/CYC"
        n89 = for {
          tunnel: w310 -> [w1835]
          tunnel: w309 -> [w1834]
          tunnel: w308 -> [w1831] mode=indexing
          tunnel: [w1826] -> w302
          tunnel: [w1830] -> w292
          n90 = local read "Set VDD"() -> (w1829:dbl)
          n91 = call "E3631A_Voltage Controller updated.vi"("VISA resource name"=w1834, "I_VDD(A)"=0.2, "Channel Controller"=w1831, "Voltage 1"=w1829, "Voltage 2"=3.3, "error in (no error)"=w1835, "Voltage 3"=-3.3) -> ("VISA resource name out"=w1830:refnum<visa-resource-name>, "error out"=w1827:errorcluster)  [unwired: 7 in]
          n92 = call "Delay T4.vi"("milliseconds to wait"=u32 100, "error in (no error)"=w1827) -> ("error out"=w1826:errorcluster)  [unwired: 9 in]
        }
        n93 = local write "TTime Completed"(w289) -> ()
        n94 = local write "Total Time"(w289) -> ()
        n95 = call "WSVCAP SHL Host TL RFFE Write - Multiple DUTs - Common Data.vi"("Data Out"="074000", "error in"=w302) -> ("error out"=w303:errorcluster)  [unwired: 13 in]
        n96 = local read "IDD Brd(uA)"() -> (w276:string)
        n97 = call "Delay T4.vi"("milliseconds to wait"=w268, "error in (no error)"=w303) -> ("error out"=w301:errorcluster)  [unwired: 9 in]
        n98 = Number To Fractional String(number="Set VDD", precision (6)=i16 2) -> (F-format string=w282:string)  [unwired: 2 in]
        n99 = call "Ke2000 Single Reading.vi"("error in (no error)"=w301, "VISA resource name"=w300) -> ("error out"=w278:errorcluster, "VISA resource name out"=w299:refnum<visa-resource-name>, "uA"=w280:string)  [unwired: 5 in, 2 out]
        n100 = call "Substration.vi"("error in (no error)"=w278, "Input2"=w276, "Input1"=w280) -> ("error out"=w277:errorcluster, "In1 - In2"=w279:string)  [unwired: 7 in]
        "IDD Stdby(uA)" <- w279
        n101 = call "WSVCAP SHL Host TL RFFE Write - Multiple DUTs - Common Data.vi"("Data Out"="074040", "error in"=w277) -> ("error out"=w263:errorcluster)  [unwired: 13 in]
        n102 = call "Delay T4.vi"("milliseconds to wait"=w268, "error in (no error)"=w263) -> ("error out"=w286:errorcluster)  [unwired: 9 in]
        n103 = case shown="True" w259 {
          tunnel: w286 -> [w333 w334]
          tunnel: [w332 w335] -> w284
          tunnel: ["DVA OFF" ("Data Out") "DVA ON" ("Data Out")] -> w285
          frame False {
            n104 = call "WSVCAP SHL Host TL RFFE Write - Multiple DUTs - Common Data.vi"("Data Out"="074820", "error in"=w333) -> ("error out"=w332:errorcluster)  [unwired: 13 in]
          }
          frame True {
            n105 = call "WSVCAP SHL Host TL RFFE Write - Multiple DUTs - Common Data.vi"("Data Out"="074800", "error in"=w334) -> ("error out"=w335:errorcluster)  [unwired: 13 in]
          }
        }
        n106 = for {
          N: 16 -> [_]
          tunnel: "Serial Number" -> [w316]
          tunnel: [w314] -> w265 mode=indexing
          i -> [w313]
          n107 = Increment(x=w313) -> (x+1=w312:i32)
          n108 = Index Array(array=w316, index (row)=w312, index (col)=1 ("disabled index (col)")) -> (element=w314:string)
        }
        n109 = case shown="True" w261 {
          tunnel: [1 ("X Repeat") w339] -> w291
          frame False {
          }
          frame True {
            n110 = local read "X Repeat"() -> (w339:i32)
          }
        }
        n111 = Not(x=w256) -> (.not. x?=w264:bool)
        n112 = call "Delay T4.vi"("milliseconds to wait"=w268, "error in (no error)"=w284) -> ("error out"=w271:errorcluster)  [unwired: 9 in]
        n113 = case shown="True" w260 {
          tunnel: w271 -> [w320 w322]
          tunnel: [w317 w321] -> w270
          tunnel: ["CAL OFF" ("Data Out") "CAL ON" ("Data Out")] -> w272
          frame False {
            n114 = call "WSVCAP SHL Host TL RFFE Write - Multiple DUTs - Common Data.vi"("Data Out"="074044", "error in"=w320) -> ("error out"=w317:errorcluster)  [unwired: 13 in]
          }
          frame True {
            n115 = for {
              tunnel: string[] ["074920", "074900"] -> [w329] mode=indexing
              tunnel: w322 -> [w326]
              tunnel: [w325] -> w321
              n116 = call "WSVCAP SHL Host TL RFFE Write - Multiple DUTs - Common Data.vi"("Data Out"=w329, "error in"=w326) -> ("error out"=w328:errorcluster)  [unwired: 13 in]
              n117 = call "Delay T4.vi"("milliseconds to wait"=u32 10, "error in (no error)"=w328) -> ("error out"=w325:errorcluster)  [unwired: 9 in]
            }
          }
        }
        n118 = for {
          N: w291 -> [_]
          tunnel: w311 -> [w378]
          tunnel: [w374] -> w307
          tunnel: [w373] -> w305
          tunnel: w279 -> [w372]
          tunnel: w299 -> [w371]
          tunnel: "TMN DC\\CAP Data Log File Path" -> [w370]
          tunnel: w297 -> [w368]
          tunnel: [w367] -> w295
          tunnel: w292 -> [w366]
          shift-right: [w361] -> _
          shift-left: u64 0 -> [w363]
          tunnel: w261 -> [w360]
          tunnel: w288 -> [w356]
          tunnel: w288 -> [w355]
          tunnel: w285 -> [w354]
          tunnel: w282 -> [w353]
          tunnel: [w352] -> w275
          tunnel: w272 -> [w351]
          tunnel: w270 -> [w350]
          tunnel: w259 -> [w349]
          tunnel: w262 -> [w347]
          tunnel: w258 -> [w346]
          tunnel: w264 -> [w345]
          tunnel: w257 -> [w344]
          tunnel: w265 -> [w343]
          tunnel: w255 -> [w342]
          tunnel: w254 -> [w341]
          tunnel: [w340] -> w253
          i -> [w359]
          stop <- w348 stop-if-true
          n119 = while {
            tunnel: w378 -> [w604]
            tunnel: w370 -> [w615]
            tunnel: "Lot#" -> [w614]
            tunnel: "Wafer#" -> [w613]
            tunnel: w343 -> [w612]
            tunnel: "Test Program" -> [w611]
            tunnel: w343 -> [w610]
            tunnel: "Comment" -> [w609]
            tunnel: "Lot#" -> [w608]
            tunnel: "Wafer#" -> [w607]
            tunnel: w371 -> [w603]
            tunnel: [w606] -> w374
            tunnel: [w596] -> w373
            tunnel: w372 -> [w602]
            tunnel: w368 -> [w599]
            tunnel: [w598] -> w367
            tunnel: w366 -> [w597]
            tunnel: [w503] -> w340
            tunnel: w359 -> [w541]
            tunnel: [w532] -> w361
            tunnel: w363 -> [w531]
            shift-right: [w530] -> _
            shift-left: u64 0 -> [w424]
            tunnel: [w529] -> w357
            tunnel: w360 -> [w527]
            tunnel: w356 -> [w502]
            tunnel: w355 -> [w500]
            tunnel: w354 -> [w448]
            tunnel: w353 -> [w446]
            tunnel: [w421] -> w352
            tunnel: w351 -> [w428]
            tunnel: w350 -> [w427]
            tunnel: w349 -> [w426]
            tunnel: w347 -> [w418]
            tunnel: w346 -> [w417]
            tunnel: w345 -> [w412]
            tunnel: w344 -> [w406]
            tunnel: w342 -> [w380]
            tunnel: w341 -> [w379]
            i -> [w528]
            stop <- w542 stop-if-true
            n120 = case shown="4" "CP to HD/Cycle" {
              selector: "CP to HD/Cycle" -> [w619 w624 w629 w634 w638]
              tunnel: string[] ["07476F", "074776", "074765", "074769", "07477B"] -> [w620 w625 w630 w635 w640]
              tunnel: [w618 w623 w628 w633 w639] -> w443
              tunnel: ["35.0" ("Data Out") "27.5" ("Data Out") "30.5" ("Data Out") "44.0" ("Data Out") "40.25" ("Data Out")] -> w442
              tunnel: [w616 w621 w626 w631 w636] -> w441
              tunnel: w427 -> [w616 w621 w626 w631 w636]
              frame 0, Default {
                n121 = Index Array(array=w620, index=w619) -> (element=w618:string)
              }
              frame 2 {
                n122 = Index Array(array=w625, index=w624) -> (element=w623:string)
              }
              frame 3 {
                n123 = Index Array(array=w630, index=w629) -> (element=w628:string)
              }
              frame 4 {
                n124 = Index Array(array=w635, index=w634) -> (element=w633:string)
              }
              frame 1 {
                n125 = Index Array(array=w640, index=w638) -> (element=w639:string)
              }
            }
            n126 = flat-sequence {
              tunnel: [w708] -> w595
              tunnel: [w653] -> w594
              tunnel: w604 -> [w706]
              tunnel: [w705] -> w593
              tunnel: w603 -> [w682]
              tunnel: w602 -> [w704]
              tunnel: [w704] -> w592
              tunnel: [w647] -> w591
              tunnel: [w650] -> w590
              tunnel: w441 -> [w695]
              tunnel: [w662] -> w589
              tunnel: w597 -> [w702]
              tunnel: [w670] -> w596
              tunnel: w541 -> [w700]
              tunnel: w528 -> [w672]
              tunnel: [w672] -> w538
              tunnel: w528 -> [w699]
              tunnel: w527 -> [w697]
              tunnel: [w696] -> w526
              tunnel: [w658] -> w521
              tunnel: [w657] -> w520
              tunnel: [w656] -> w519
              tunnel: [w661] -> w509
              tunnel: [w659] -> w508
              tunnel: w502 -> [w694]
              tunnel: [w694] -> w501
              tunnel: w500 -> [w693]
              tunnel: [w660] -> w487
              tunnel: [w655] -> w461
              tunnel: [w692] -> w449
              tunnel: w443 -> [w690]
              tunnel: [w674] -> w440
              tunnel: [w673] -> w432
              tunnel: w418 -> [w666]
              tunnel: w417 -> [w665]
              tunnel: [w665] -> w416
              tunnel: w412 -> [w664]
              tunnel: [w664] -> w411
              tunnel: w406 -> [w663]
              tunnel: [w663] -> w405
              tunnel: ["WS1050/51"] -> w398
              tunnel: ["Test Sequences"] -> w388
              tunnel: "Real No. From\nLookup Table" -> [w644]
              tunnel: ["Cmin/Act"] -> w384
              tunnel: w380 -> [w642]
              tunnel: w379 -> [w641]
              tunnel: w595 -> [w1022]
              tunnel: [w1018] -> w499
              tunnel: w594 -> [w1021]
              tunnel: w593 -> [w1028]
              tunnel: [w1028] -> w498
              tunnel: w592 -> [w1027]
              tunnel: w591 -> [w1020]
              tunnel: w590 -> [w1019]
              tunnel: [w1005] -> w497
              tunnel: [w1027] -> w496
              tunnel: [w1020] -> w495
              tunnel: [w1019] -> w494
              tunnel: w589 -> [w1025]
              tunnel: w538 -> [w1024]
              tunnel: [w1024] -> w493
              tunnel: w526 -> [w1023]
              tunnel: [w1023] -> w492
              tunnel: [w1021] -> w491
              tunnel: w521 -> [w1016]
              tunnel: w520 -> [w1010]
              tunnel: w519 -> [w1008]
              tunnel: [w1013] -> w490
              tunnel: w509 -> [w1015]
              tunnel: w508 -> [w1013]
              tunnel: [w1006] -> w489
              tunnel: w501 -> [w1014]
              tunnel: [w1011] -> w488
              tunnel: w487 -> [w1011]
              tunnel: [w1010] -> w486
              tunnel: w461 -> [w1009]
              tunnel: [w1009] -> w460
              tunnel: [w1008] -> w458
              tunnel: w449 -> [w1012]
              tunnel: [w1007] -> w433
              tunnel: w432 -> [w1007]
              tunnel: w416 -> [w1004]
              tunnel: [w1004] -> w415
              tunnel: w411 -> [w1003]
              tunnel: [w1003] -> w410
              tunnel: w405 -> [w1002]
              tunnel: [w1002] -> w404
              tunnel: w398 -> [w998]
              tunnel: [w998] -> w397
              tunnel: w388 -> [w997]
              tunnel: [w997] -> w387
              tunnel: w384 -> [w996]
              tunnel: [w996] -> w383
              tunnel: w499 -> [w1133]
              tunnel: [w1132] -> w485
              tunnel: w498 -> [w1146]
              tunnel: [w1146] -> w482
              tunnel: w497 -> [w1145]
              tunnel: [w1145] -> w480
              tunnel: w496 -> [w1144]
              tunnel: [w1144] -> w478
              tunnel: w495 -> [w1143]
              tunnel: [w1143] -> w476
              tunnel: w494 -> [w1142]
              tunnel: [w1142] -> w474
              tunnel: w493 -> [w1141]
              tunnel: [w1141] -> w472
              tunnel: w492 -> [w1140]
              tunnel: [w1140] -> w470
              tunnel: w491 -> [w1139]
              tunnel: [w1139] -> w468
              tunnel: w490 -> [w1138]
              tunnel: [w1138] -> w466
              tunnel: [w1127] -> w464
              tunnel: w489 -> [w1126]
              tunnel: w488 -> [w1136]
              tunnel: w486 -> [w1134]
              tunnel: w460 -> [w1131]
              tunnel: [w1131] -> w459
              tunnel: w458 -> [w1130]
              tunnel: [w1130] -> w457
              tunnel: [w1128] -> w456
              tunnel: [w1129] -> w434
              tunnel: w433 -> [w1129]
              tunnel: w415 -> [w1125]
              tunnel: [w1125] -> w414
              tunnel: w410 -> [w1124]
              tunnel: [w1124] -> w409
              tunnel: w404 -> [w1123]
              tunnel: [w1123] -> w403
              tunnel: w397 -> [w1122]
              tunnel: [w1122] -> w396
              tunnel: w387 -> [w1121]
              tunnel: [w1121] -> w386
              tunnel: w383 -> [w1120]
              tunnel: [w1120] -> w382
              tunnel: w485 -> [w1220]
              tunnel: [w1219] -> w484
              tunnel: [w1215] -> w483
              tunnel: w482 -> [w1232]
              tunnel: [w1232] -> w481
              tunnel: w480 -> [w1231]
              tunnel: [w1231] -> w479
              tunnel: w478 -> [w1230]
              tunnel: [w1230] -> w477
              tunnel: w476 -> [w1229]
              tunnel: [w1229] -> w475
              tunnel: w474 -> [w1228]
              tunnel: [w1228] -> w473
              tunnel: w472 -> [w1227]
              tunnel: [w1227] -> w471
              tunnel: w470 -> [w1226]
              tunnel: [w1226] -> w469
              tunnel: w468 -> [w1225]
              tunnel: [w1225] -> w467
              tunnel: w466 -> [w1224]
              tunnel: [w1224] -> w465
              tunnel: w464 -> [w1223]
              tunnel: [w1223] -> w463
              tunnel: [w1213] -> w462
              tunnel: w459 -> [w1222]
              tunnel: w457 -> [w1221]
              tunnel: w456 -> [w1214]
              tunnel: [w1218] -> w447
              tunnel: [w1217] -> w435
              tunnel: w434 -> [w1217]
              tunnel: w426 -> [w1216]
              tunnel: [w1216] -> w425
              tunnel: w414 -> [w1212]
              tunnel: [w1212] -> w413
              tunnel: w409 -> [w1211]
              tunnel: [w1211] -> w408
              tunnel: w403 -> [w1210]
              tunnel: [w1210] -> w402
              tunnel: w396 -> [w1209]
              tunnel: [w1209] -> w395
              tunnel: [w1209] -> w393
              tunnel: [w1209] -> w392
              tunnel: w386 -> [w1208]
              tunnel: w382 -> [w1207]
              tunnel: [w1207] -> w381
              tunnel: [w1360] -> w588
              tunnel: [w1326] -> w587
              tunnel: w484 -> [w1364]
              tunnel: w483 -> [w1340]
              tunnel: [w1349] -> w586
              tunnel: [w1340] -> w585
              tunnel: [w1363] -> w584
              tunnel: [w1362] -> w583
              tunnel: w481 -> [w1361]
              tunnel: [w1361] -> w582
              tunnel: w479 -> [w1349]
              tunnel: w477 -> [w1359]
              tunnel: [w1359] -> w581
              tunnel: w475 -> [w1355]
              tunnel: [w1355] -> w580
              tunnel: w473 -> [w1354]
              tunnel: [w1354] -> w579
              tunnel: w471 -> [w1350]
              tunnel: [w1350] -> w537
              tunnel: w469 -> [w1358]
              tunnel: [w1358] -> w525
              tunnel: w467 -> [w1357]
              tunnel: [w1356] -> w522
              tunnel: w465 -> [w1352]
              tunnel: w463 -> [w1348]
              tunnel: [w1353] -> w518
              tunnel: [w1351] -> w517
              tunnel: [w1348] -> w512
              tunnel: w462 -> [w1347]
              tunnel: [w1334] -> w507
              tunnel: [w1333] -> w506
              tunnel: [w1332] -> w505
              tunnel: w447 -> [w1346]
              tunnel: [w1331] -> w436
              tunnel: w435 -> [w1331]
              tunnel: [w1330] -> w431
              tunnel: w425 -> [w1329]
              tunnel: w413 -> [w1324]
              tunnel: w408 -> [w1323]
              tunnel: [w1323] -> w407
              tunnel: w402 -> [w1322]
              tunnel: [w1322] -> w401
              tunnel: w395 -> [w1312]
              tunnel: [w1312] -> w394
              tunnel: w393 -> [w1311]
              tunnel: w392 -> [w1310]
              tunnel: w381 -> [w1309]
              tunnel: w588 -> [w1583]
              tunnel: [w1583] -> w578
              tunnel: [w1568] -> w577
              tunnel: [w1582] -> w576
              tunnel: w587 -> [w1581]
              tunnel: w586 -> [w1580]
              tunnel: w585 -> [w1579]
              tunnel: [w1580] -> w575
              tunnel: [w1579] -> w574
              tunnel: w584 -> [w1578]
              tunnel: [w1578] -> w573
              tunnel: w583 -> [w1577]
              tunnel: [w1577] -> w572
              tunnel: w582 -> [w1576]
              tunnel: [w1576] -> w571
              tunnel: w581 -> [w1575]
              tunnel: [w1575] -> w570
              tunnel: w580 -> [w1574]
              tunnel: [w1574] -> w569
              tunnel: w579 -> [w1573]
              tunnel: [w1573] -> w568
              tunnel: w599 -> [w1572]
              tunnel: [w1570] -> w567
              tunnel: [w1550] -> w566
              tunnel: [w1551] -> w565
              tunnel: [w1549] -> w564
              tunnel: w537 -> [w1566]
              tunnel: [w1566] -> w536
              tunnel: w525 -> [w1565]
              tunnel: [w1565] -> w524
              tunnel: w522 -> [w1582]
              tunnel: w518 -> [w1563]
              tunnel: w517 -> [w1564]
              tunnel: [w1564] -> w516
              tunnel: [w1563] -> w514
              tunnel: w512 -> [w1562]
              tunnel: [w1562] -> w511
              tunnel: w507 -> [w1548]
              tunnel: w506 -> [w1547]
              tunnel: w505 -> [w1546]
              tunnel: [w1543] -> w504
              tunnel: [w1548] -> w455
              tunnel: [w1547] -> w453
              tunnel: [w1546] -> w451
              tunnel: [w1545] -> w437
              tunnel: w436 -> [w1545]
              tunnel: w431 -> [w1544]
              tunnel: [w1544] -> w430
              tunnel: w407 -> [w1543]
              tunnel: w401 -> [w1542]
              tunnel: w394 -> [w1541]
              tunnel: [w1541] -> w391
              tunnel: w578 -> [w1677]
              tunnel: [w1677] -> w563
              tunnel: w577 -> [w1701]
              tunnel: [w1700] -> w562
              tunnel: w615 -> [w1702]
              tunnel: w614 -> [w1699]
              tunnel: w613 -> [w1698]
              tunnel: w612 -> [w1697]
              tunnel: [w1696] -> w561
              tunnel: w576 -> [w1690]
              tunnel: [w1690] -> w560
              tunnel: w575 -> [w1695]
              tunnel: w574 -> [w1694]
              tunnel: [w1695] -> w559
              tunnel: [w1694] -> w558
              tunnel: [w1685] -> w557
              tunnel: w573 -> [w1693]
              tunnel: [w1693] -> w556
              tunnel: w572 -> [w1692]
              tunnel: [w1692] -> w555
              tunnel: w571 -> [w1689]
              tunnel: [w1691] -> w554
              tunnel: w424 -> [w1688]
              tunnel: [w1687] -> w553
              tunnel: [w1675] -> w552
              tunnel: w570 -> [w1686]
              tunnel: w569 -> [w1684]
              tunnel: w568 -> [w1683]
              tunnel: "File Name" -> [w1682]
              tunnel: w567 -> [w1681]
              tunnel: [w1681] -> w551
              tunnel: w566 -> [w1680]
              tunnel: [w1680] -> w550
              tunnel: [w1679] -> w549
              tunnel: w565 -> [w1679]
              tunnel: w564 -> [w1678]
              tunnel: [w1678] -> w548
              tunnel: [w1673] -> w539
              tunnel: w536 -> [w1674]
              tunnel: [w1674] -> w534
              tunnel: w531 -> [w1672]
              tunnel: w524 -> [w1671]
              tunnel: [w1671] -> w523
              tunnel: w516 -> [w1670]
              tunnel: [w1670] -> w515
              tunnel: w514 -> [w1669]
              tunnel: [w1669] -> w513
              tunnel: w511 -> [w1668]
              tunnel: [w1668] -> w510
              tunnel: w504 -> [w1667]
              tunnel: w455 -> [w1666]
              tunnel: [w1666] -> w454
              tunnel: w453 -> [w1665]
              tunnel: [w1665] -> w452
              tunnel: w451 -> [w1664]
              tunnel: [w1664] -> w450
              tunnel: w440 -> [w1663]
              tunnel: [w1663] -> w439
              tunnel: [w1662] -> w438
              tunnel: w437 -> [w1662]
              tunnel: w430 -> [w1661]
              tunnel: [w1661] -> w429
              tunnel: ["Freq(Hz)"] -> w400
              tunnel: ["Brd #"] -> w399
              tunnel: w391 -> [w1658]
              tunnel: [w1658] -> w390
              tunnel: w563 -> [w1772]
              tunnel: w562 -> [w1771]
              tunnel: w615 -> [w1734]
              tunnel: w611 -> [w1766]
              tunnel: w610 -> [w1769]
              tunnel: w609 -> [w1765]
              tunnel: w608 -> [w1768]
              tunnel: w607 -> [w1764]
              tunnel: w561 -> [w1767]
              tunnel: [w1772] -> w544
              tunnel: [w1770] -> w545
              tunnel: w560 -> [w1762]
              tunnel: [w1762] -> w546
              tunnel: w559 -> [w1761]
              tunnel: w558 -> [w1746]
              tunnel: w557 -> [w1760]
              tunnel: w556 -> [w1759]
              tunnel: w555 -> [w1748]
              tunnel: [w1756] -> w547
              tunnel: w554 -> [w1758]
              tunnel: w553 -> [w1757]
              tunnel: w552 -> [w1756]
              tunnel: "File Name" -> [w1727]
              tunnel: w551 -> [w1755]
              tunnel: [w1755] -> w543
              tunnel: w550 -> [w1754]
              tunnel: w549 -> [w1753]
              tunnel: w548 -> [w1752]
              tunnel: [w1751] -> w540
              tunnel: w539 -> [w1751]
              tunnel: [w1730] -> w535
              tunnel: w534 -> [w1730]
              tunnel: w523 -> [w1750]
              tunnel: w515 -> [w1749]
              tunnel: w513 -> [w1747]
              tunnel: w510 -> [w1745]
              tunnel: w454 -> [w1744]
              tunnel: w452 -> [w1743]
              tunnel: w450 -> [w1742]
              tunnel: w448 -> [w1741]
              tunnel: w428 -> [w1740]
              tunnel: w442 -> [w1739]
              tunnel: w446 -> [w1738]
              tunnel: w439 -> [w1737]
              tunnel: w438 -> [w1736]
              tunnel: w429 -> [w1735]
              tunnel: [w1732] -> w423
              tunnel: [w1723] -> w419
              tunnel: w400 -> [w1722]
              tunnel: w399 -> [w1721]
              tunnel: w390 -> [w1720]
              tunnel: [w1720] -> w389
              tunnel: [w1794] -> w605
              tunnel: [w1795] -> w606
              tunnel: [w1796] -> w503
              tunnel: w547 -> [w1787]
              tunnel: w546 -> [w1795]
              tunnel: w545 -> [w1782]
              tunnel: w544 -> [w1796]
              tunnel: w543 -> [w1789]
              tunnel: [w1789] -> w598
              tunnel: [w1786] -> w532
              tunnel: w540 -> [w1786]
              tunnel: w535 -> [w1788]
              tunnel: [w1788] -> w533
              tunnel: [w1787] -> w530
              tunnel: [w1785] -> w529
              tunnel: [w1781] -> w420
              tunnel: w423 -> [w1780]
              tunnel: w419 -> [w1778]
              tunnel: w389 -> [w1777]
              frame #0 {
                n127 = call "WSVCAP SHL Host TL RFFE Write - Multiple DUTs - Common Data.vi"("Data Out"=w690, "error in"=w695) -> ("error out"=w668:errorcluster)  [unwired: 13 in]
                n128 = Index Array(array=w706, index (row)=w699, index (col)=0 ("disabled index (col)")) -> (element=w698:dbl)
                n129 = for {
                  tunnel: string[] ["0760", "0767", "0768"] -> [w753] mode=indexing
                  tunnel: [w749] -> w679 mode=indexing
                  tunnel: w668 -> [w747]
                  tunnel: [w746] -> w671
                  i -> [w752]
                  n130 = call "Delay T4.vi"("milliseconds to wait"=u32 10, "error in (no error)"=w747) -> ("error out"=w754:errorcluster)  [unwired: 9 in]
                  n131 = call "WSVCAP SHL Host TL RFFE Read - Multiple DUTs - Common Data.vi"("Data Out"=w753, "error in"=w754) -> ("RFFE Data In"=w751:string[], "error out"=w746:errorcluster)  [unwired: 12 in]
                  n132 = Index Array(array=w751, index=w752) -> (element=w748:string)
                  n133 = String Subset(string=w748, offset (0)=0) -> (substring=w749:string)  [unwired: 1 in]
                }
                "RB Reg for HD/Cycle" <- w679
                n134 = call "Delay T4.vi"("milliseconds to wait"=u32 100, "error in (no error)"=w671) -> ("error out"=w685:errorcluster)  [unwired: 9 in]
                n135 = local read "IDD Brd(uA)"() -> (w689:string)
                n136 = call "Ke2000 Single Reading.vi"("error in (no error)"=w685, "VISA resource name"=w682) -> ("error out"=w687:errorcluster, "VISA resource name out"=w681:refnum<visa-resource-name>, "uA"=w688:string)  [unwired: 5 in, 2 out]
                n137 = call "Substration.vi"("error in (no error)"=w687, "Input2"=w689, "Input1"=w688) -> ("error out"=w684:errorcluster, "In1 - In2"=→"IDD_HD/CYC (uA)":string)  [unwired: 7 in]
                n138 = case shown="False" w697 {
                  tunnel: [w786 w883] -> w708
                  tunnel: [w787 w868] -> w703
                  tunnel: [w785 w885] -> w705
                  tunnel: w684 -> [w781 w872]
                  tunnel: w702 -> [w777 w884]
                  tunnel: [w777 w884] -> w670
                  tunnel: w700 -> [_ w874]
                  tunnel: w698 -> [w778 w869]
                  tunnel: [w783 w870] -> w696
                  tunnel: w672 -> [w769 w866]
                  tunnel: w693 -> [w780 _]
                  tunnel: ["%Duty Cycle" "100" ("Data Out")] -> w674
                  tunnel: w666 -> [w767 _]
                  tunnel: w644 -> [w766 w859]
                  tunnel: w642 -> [w763 _]
                  tunnel: w641 -> [w762 _]
                  frame False {
                    # "Cycles in 1s"
                    n139 = case shown="False" w766 {
                      tunnel: w781 -> [w793 w799]
                      tunnel: w778 -> [w792 w798]
                      tunnel: [w791 w799] -> w776
                      tunnel: w769 -> [w790 _]
                      tunnel: [w789 w798] -> w775
                      tunnel: [u64 1000 ("y") u64 1 ("y")] -> w770
                      frame False {
                        n140 = case shown="8, Default" w790 {
                          tunnel: w792 -> [w795 _]
                          tunnel: [w795 "CYC RP (X1000)"] -> w789
                          tunnel: [w794 w796] -> w791
                          tunnel: w793 -> [w794 w796]
                          frame 0..7 {
                          }
                          frame 8, Default {
                          }
                        }
                      }
                      frame True {
                        # "Read real number\nfrom lookup table"
                      }
                    }
                    n141 = call "WSVCAP SHL Host TL RFFE Configure.vi"("RFFE Slave Address"=w780, "Clock Rate (Hz)"="SPI Clock Rate (Hz)", "error in"=w776) -> ("Actual Rate (Hz)"=→"AR Cycling(Hz)":dbl, "error out"=w764:errorcluster)  [unwired: 11 in]
                    n142 = Array Max & Min(array=w762) -> (max value=w773:dbl)  [unwired: 3 out]
                    n143 = Divide(x=1.0, y=w773) -> (x/y=w772:dbl)
                    n144 = To Unsigned Quad Integer(1:w772) -> (0:w771:u64)
                    n145 = Not(x=w767) -> (.not. x?=w768:bool)
                    n146 = case shown="True" w768 {
                      tunnel: [w802 w824] -> w787
                      tunnel: [w805 w823] -> w786
                      tunnel: [u64 1 w822] -> w785
                      tunnel: w764 -> [w803 w821]
                      tunnel: w775 -> [_ w820]
                      tunnel: w762 -> [_ w818]
                      tunnel: w771 -> [_ w817]
                      tunnel: w770 -> [_ w816]
                      tunnel: w769 -> [w801 _]
                      tunnel: w763 -> [_ w815]
                      frame False {
                        n147 = case shown="1, Default" w801 {
                          tunnel: w803 -> [w806 w808]
                          tunnel: [w806 w807] -> w802
                          frame 0 {
                          }
                          frame 1, Default {
                            n148 = flat-sequence {
                              tunnel: "Repeat Meas(s)" -> [w814]
                              tunnel: w808 -> [w811]
                              tunnel: [w811] -> w807
                              frame #0 {
                                n149 = Multiply(x=w814, y=u32 1000) -> (x*y=w813:u32)
                                n150 = Wait (ms)(milliseconds to wait=w813) -> ()  [unwired: 1 out]
                                n151 = local write "STATUS"("Verify Sockets waiting times..." ("STATUS")) -> ()
                              }
                            }
                          }
                        }
                        n152 = local read "stop During HD/Cycles"() -> (w805:bool)
                      }
                      frame True {
                        n153 = while {
                          tunnel: w820 -> [w844]
                          tunnel: [w831] -> w824
                          tunnel: [w836] -> w823
                          tunnel: w821 -> [w842]
                          tunnel: [w830] -> w822
                          tunnel: w815 -> [w841]
                          tunnel: w818 -> [w840]
                          tunnel: w817 -> [w827]
                          tunnel: w816 -> [w825]
                          i -> [w839]
                          stop <- w835 stop-if-true
                          # "At least 1 second before target"
                          # "Remaining Cycles"
                          # "Target Cycles"
                          # "Cycles in 1s"
                          n154 = To Unsigned Quad Integer(1:w844) -> (0:w843:u64)
                          n155 = case shown="0" w839 {
                            tunnel: [w851 w853] -> w833
                            tunnel: w842 -> [w852 w853]
                            tunnel: w841 -> [w850 _]
                            tunnel: w840 -> [w849 _]
                            frame 0 {
                              n156 = call "WSVCAP SHL Host TL RFFE Write Cycle - Multiple DUTs - Common Data1.vi"("Data Out (Cycle Commands)"=w850, "Post Command Delay"=w849, "error in"=w852) -> ("error out"=w851:errorcluster)  [unwired: 12 in]
                            }
                            frame 1, Default {
                            }
                          }
                          n157 = Multiply(x=w843, y=w825) -> (x*y=w830:u64)
                          n158 = call "WSVCAP SHL Host TL SPI_RFFE Query Cycle Count.vi"("error in"=w833) -> ("Cycle Count"=w829:u64, "error out"=w838:errorcluster)  [unwired: 13 in]
                          "Cycle Count" <- w829
                          n159 = Subtract(x=w830, y=w829) -> (x-y=w828:u64)
                          n160 = Greater Or Equal?(x=w829, y=w830) -> (x >= y?=w837:bool)
                          n161 = local read "stop During HD/Cycles"() -> (w836:bool)
                          n162 = Greater?(x=w828, y=w827) -> (0:w826:bool)
                          n163 = case shown="True" w837 {
                            tunnel: [w855 w858] -> w832
                            tunnel: w838 -> [w855 w857]
                            tunnel: [FALSE TRUE] -> w834
                            frame False {
                            }
                            frame True {
                              n164 = call "WSVCAP SHL Host TL RFFE Stop Write Cycle.vi"("error in"=w857) -> ("error out"=w858:errorcluster)  [unwired: 14 in]
                            }
                          }
                          n165 = Or(x=w834, y=w836) -> (x .or. y?=w835:bool)
                          n166 = case shown="True" w826 {
                            tunnel: w832 -> [w845 w848]
                            tunnel: [w845 w847] -> w831
                            frame False {
                            }
                            frame True {
                              n167 = call "MISC Wait with Data Flow.vi"("Error In (no error)"=w848, "Wait Time (500ms)"=u32 50) -> ("Error Out"=w847:errorcluster)  [unwired: 7 in, 2 out]
                            }
                          }
                        }
                        n168 = local write "STATUS"("Parts are Cycling...." ("STATUS")) -> ()
                      }
                    }
                    n169 = local read "HD/CYC Temp"() -> (w782:i32)
                    n170 = Number To Engineering String(4:w782) -> (0:w783:string)  [unwired: 3 in]
                  }
                  frame True {
                    n171 = case shown="False" w859 {
                      tunnel: w874 -> [w891 _]
                      tunnel: [w890 w903] -> w873
                      tunnel: w872 -> [w889 w904]
                      tunnel: [w888 w904] -> w871
                      tunnel: w869 -> [w887 w903]
                      tunnel: w866 -> [w886 _]
                      frame False {
                        n172 = case shown="0" w891 {
                          tunnel: [w894 w901] -> w890
                          tunnel: w889 -> [w896 w902]
                          tunnel: [w895 w902] -> w888
                          tunnel: w887 -> [w893 _]
                          tunnel: w886 -> [w892 _]
                          frame 0 {
                            n173 = case shown="15, Default" w892 {
                              tunnel: [w897 "HD RP(Min)"] -> w894
                              tunnel: w896 -> [w898 w900]
                              tunnel: [w898 w900] -> w895
                              tunnel: w893 -> [w897 _]
                              frame 0..14 {
                              }
                              frame 15, Default {
                              }
                            }
                          }
                          frame 1, Default {
                            n174 = local read "HD RP(Min)"() -> (w901:dbl)
                          }
                        }
                      }
                      frame True {
                      }
                    }
                    n175 = flat-sequence {
                      tunnel: [w978] -> w879
                      tunnel: w871 -> [w984]
                      frame #0 {
                        n176 = call "WSVCAP SHL Host TL RFFE Write - Multiple DUTs - Common Data.vi"("Data Out"="Cmd to HD", "error in"=w984) -> ("error out"=w983:errorcluster)  [unwired: 13 in]
                        n177 = call "Delay T4.vi"("milliseconds to wait"=u32 50, "error in (no error)"=w983) -> ("error out"=w980:errorcluster)  [unwired: 9 in]
                        n178 = for {
                          tunnel: string[] ["0761", "0762", "0763"] -> [w995] mode=indexing
                          tunnel: [w991] -> w979 mode=indexing
                          shift-right: [w988] -> w978
                          shift-left: w980 -> [w994]
                          i -> [w993]
                          n179 = call "WSVCAP SHL Host TL RFFE Read - Multiple DUTs - Common Data.vi"("Data Out"=w995, "error in"=w994) -> ("RFFE Data In"=w990:string[], "error out"=w987:errorcluster)  [unwired: 12 in]
                          n180 = Index Array(array=w990, index=w993) -> (element=w989:string)
                          n181 = call "Delay T4.vi"("milliseconds to wait"=u32 10, "error in (no error)"=w987) -> ("error out"=w988:errorcluster)  [unwired: 9 in]
                          n182 = String Subset(string=w989, offset (0)=0) -> (substring=w991:string)  [unwired: 1 in]
                        }
                        "RB Reg for HD" <- w979
                      }
                    }
                    n183 = local read "No of HD/Cycle\nCompleted"() -> (w875:u64)
                    n184 = Greater?(x="HD_DC (Min)", y=w875) -> (0:w876:bool)
                    n185 = case shown="True" w876 {
                      tunnel: [_ w911] -> w881
                      tunnel: [w906 w910] -> w880
                      tunnel: w879 -> [w906 w909]
                      tunnel: w873 -> [w905 w908]
                      tunnel: [w905 w907] -> w878
                      frame False {
                      }
                      frame True {
                        n186 = flat-sequence {
                          tunnel: [w916] -> w911
                          tunnel: [w915] -> w910
                          tunnel: w909 -> [w914]
                          tunnel: w908 -> [w912]
                          tunnel: [w912] -> w907
                          frame #0 {
                            # "HD"
                            n187 = Multiply(x=1000.0, y=w912) -> (x*y=w919:dbl)
                            n188 = Multiply(x=60.0, y=w919) -> (x*y=w917:dbl)
                            n189 = local write "STATUS"("Parts are Holding Down..." ("STATUS")) -> ()
                            n190 = event shown="[0] Timeout" {
                              selector: _ -> [_ _]
                              dyn-events: _ -> [_ _]
                              timeout: w917 -> [_ _]
                              tunnel: ["stop During HD/Cycles" TRUE ("stop During HD/Cycles")] -> w916
                              tunnel: w914 -> [w921 w923]
                              tunnel: [w921 w923] -> w915
                              event Timeout {
                                n191 = event-data() -> ()  [unwired: 1 in, 2 out]
                              }
                              event "stop During HD/Cycles": Value Change {
                                n192 = event-data() -> ()  [unwired: 1 in, 2 out]
                              }
                            }
                          }
                        }
                      }
                    }
                    n193 = Greater Or Equal?(x=w875, y="HD_DC (Min)") -> (x >= y?=w882:bool)
                    n194 = To Unsigned Quad Integer(1:w873) -> (0:w885:u64)
                    n195 = Add(x="Time All OFF (s)", y="Time All ON (s)") -> (x+y=w861:u32)
                    n196 = To Double Precision Float(number=w861) -> (double precision float=w860:dbl)
                    n197 = Divide(x=w860, y=60.0) -> (x/y=w862:dbl)
                    n198 = case shown="True" w882 {
                      tunnel: [w927 w940] -> w883
                      tunnel: [w928 w932] -> w868
                      tunnel: w880 -> [w928 w939]
                      tunnel: w881 -> [w927 w938]
                      tunnel: w878 -> [_ w937]
                      tunnel: [w926 w935] -> w870
                      tunnel: w862 -> [_ w929]
                      frame False {
                        n199 = Number To Engineering String(4:"HD/CYC Temp") -> (0:w926:string)  [unwired: 3 in]
                      }
                      frame True {
                        n200 = Divide(x=w937, y=w929) -> (x/y=w936:dbl)
                        n201 = call "WSVCAP SHL Host TL RFFE Write - Multiple DUTs - Common Data.vi"("Data Out"="070201000000", "error in"=w939) -> ("error out"=w942:errorcluster)  [unwired: 13 in]
                        n202 = Round To Nearest(number=w936) -> (nearest integer value=w931:dbl)
                        n203 = call "Delay T4.vi"("milliseconds to wait"=u32 50, "error in (no error)"=w942) -> ("error out"=w933:errorcluster)  [unwired: 9 in]
                        n204 = To Long Integer(number=w931) -> (32bit integer=w930:i32)
                        "No LPs to RP" <- w930
                        n205 = for {
                          N: w930 -> [_]
                          tunnel: w938 -> [w957]
                          tunnel: [w956] -> w940
                          tunnel: w933 -> [w945]
                          tunnel: [w944] -> w932
                          i -> [w955]
                          stop <- w956 stop-if-true
                          n206 = Increment(x=w955) -> (x+1=→"LPs Count":i32)
                          n207 = call "WSVCAP SHL Host TL RFFE Write - Multiple DUTs - Common Data.vi"("Data Out"="074776", "error in"=w945) -> ("error out"=w963:errorcluster)  [unwired: 13 in]
                          n208 = call "Delay T4.vi"("milliseconds to wait"=u32 1, "error in (no error)"=w963) -> ("error out"=w962:errorcluster)  [unwired: 9 in]
                          n209 = local read "CP to HD/Cycle"() -> (w947:i32)
                          n210 = call "WSVCAP SHL Host TL RFFE Write - Multiple DUTs - Common Data.vi"("Data Out"="070201000000", "error in"=w948) -> ("error out"=w959:errorcluster)  [unwired: 13 in]
                          n211 = call "WSVCAP SHL Host TL RFFE Write - Multiple DUTs - Common Data.vi"("Data Out"="0702013B3B3B", "error in"=w962) -> ("error out"=w952:errorcluster)  [unwired: 13 in]
                          n212 = flat-sequence {
                            tunnel: w959 -> [w971]
                            tunnel: [w969] -> w944
                            frame #0 {
                              n213 = local read "Time All OFF (s)"() -> (w966:u32)
                              n214 = local write "STATUS"("Now HD OFF Time..." ("STATUS")) -> ()
                              n215 = Multiply(x=w966, y=u32 1000) -> (x*y=w968:u32)
                              n216 = call "Delay T4.vi"("milliseconds to wait"=w968, "error in (no error)"=w971) -> ("error out"=w969:errorcluster)  [unwired: 9 in]
                            }
                          }
                          n217 = call "Delay T4.vi"("milliseconds to wait"=u32 1, "error in (no error)"=w952) -> ("error out"=w950:errorcluster)  [unwired: 9 in]
                          n218 = Index Array(array=string[] ["07476F", "074776", "074765", "074769", "07477B"], index=w947) -> (element=w953:string)
                          n219 = call "WSVCAP SHL Host TL RFFE Write - Multiple DUTs - Common Data.vi"("Data Out"=w953, "error in"=w950) -> ("error out"=w949:errorcluster)  [unwired: 13 in]
                          n220 = flat-sequence {
                            tunnel: [w976] -> w948
                            tunnel: w949 -> [w972]
                            frame #0 {
                              n221 = local read "Time All ON (s)"() -> (w973:u32)
                              n222 = local write "STATUS"("Now HD ON Time..." ("STATUS")) -> ()
                              n223 = Multiply(x=w973, y=u32 1000) -> (x*y=w975:u32)
                              n224 = call "Delay T4.vi"("milliseconds to wait"=w975, "error in (no error)"=w972) -> ("error out"=w976:errorcluster)  [unwired: 9 in]
                            }
                          }
                          n225 = Unbundle By Name(w944) -> ("status"=w958:bool)
                          n226 = Or(x=w958, y=w957) -> (x .or. y?=w956:bool)
                        }
                        n227 = Number To Engineering String(4:"DC_Temp") -> (0:w935:string)  [unwired: 3 in]
                      }
                    }
                  }
                }
                n228 = case shown="4" "CP to Meas" {
                  selector: "CP to Meas" -> [w724 w729 w734 w739 w743]
                  tunnel: string[] ["07476F", "074776", "074765", "074769", "07477B"] -> [w725 w730 w735 w740 w745]
                  tunnel: [w723 w728 w733 w738 w744] -> w677
                  tunnel: [w722 w727 w732 w737 w742] -> w667
                  tunnel: w676 -> [w722 w727 w732 w737 w742]
                  tunnel: ["35" ("Data Out") "27.5" ("Data Out") "30.5" ("Data Out") "44.0" ("Data Out") "40.25" ("Data Out")] -> w673
                  frame 0, Default {
                    n229 = Index Array(array=w725, index=w724) -> (element=w723:string)
                  }
                  frame 2 {
                    n230 = Index Array(array=w730, index=w729) -> (element=w728:string)
                  }
                  frame 3 {
                    n231 = Index Array(array=w735, index=w734) -> (element=w733:string)
                  }
                  frame 4 {
                    n232 = Index Array(array=w740, index=w739) -> (element=w738:string)
                  }
                  frame 1 {
                    n233 = Index Array(array=w745, index=w743) -> (element=w744:string)
                  }
                }
                n234 = call "WSVCAP SHL Host TL RFFE Write - Multiple DUTs - Common Data.vi"("Data Out"=w677, "error in"=w667) -> ("error out"=w691:errorcluster)  [unwired: 13 in]
                n235 = flat-sequence {
                  tunnel: w703 -> [w761]
                  tunnel: [w761] -> w676
                  frame #0 {
                    w757 = "0" ("NOM IDD OFF(uA)")
                    w758 = string[] []
                    w759 = string[][] []
                    n236 = To Long Integer(number=0.0 ("No of Loops to RP")) -> (32bit integer=w756:i32)
                    n237 = local write "LPs Count"(w756) -> ()
                    n238 = local write "No LPs to RP"(w756) -> ()
                    n239 = local write "NOM IDD ON (uA)"(w757) -> ()
                    n240 = local write "Current EFuse Read back"(w758) -> ()
                    n241 = local write "RB Reg for HD"(w758) -> ()
                    n242 = local write "RB Reg for HD/Cycle"(w758) -> ()
                    n243 = local write "NOM IDD OFF(uA)"(w757) -> ()
                    n244 = local write "Total Delta 1(pF)"(w758) -> ()
                    n245 = local write "Total Delta 2(pF)"(w758) -> ()
                    n246 = local write "Total Delta 3(pF)"(w758) -> ()
                    n247 = local write "VSA_V3"(w759) -> ()
                    n248 = local write "VSA_V1"(w759) -> ()
                    n249 = local write "VSA_V2"(w759) -> ()
                    n250 = local write "VPI C1"(w759) -> ()
                    n251 = local write "VPI C2"(w759) -> ()
                    n252 = local write "VPI C3"(w759) -> ()
                    n253 = local write "% Delta C"(w759) -> ()
                    n254 = local write "40V_3"(w759) -> ()
                    n255 = local write "40V_2"(w759) -> ()
                    n256 = local write "40V_1"(w759) -> ()
                  }
                }
                n257 = call "Delay T4.vi"("milliseconds to wait"=u32 50, "error in (no error)"=w691) -> ("error out"=w669:errorcluster)  [unwired: 9 in]
                n258 = for {
                  tunnel: [w720] -> w648 mode=indexing
                  tunnel: w681 -> [w718]
                  tunnel: w669 -> [w717]
                  tunnel: [w711] -> w653
                  tunnel: string[] ["0702013B3B3B", "070201000000"] -> [w710] mode=indexing
                  tunnel: [w709] -> w646
                  n259 = call "WSVCAP SHL Host TL RFFE Write - Multiple DUTs - Common Data.vi"("Data Out"=w710, "error in"=w717) -> ("error out"=w714:errorcluster)  [unwired: 13 in]
                  n260 = call "Delay T4.vi"("milliseconds to wait"=u32 100, "error in (no error)"=w714) -> ("error out"=w715:errorcluster)  [unwired: 9 in]
                  n261 = local read "IDD Brd(uA)"() -> (w719:string)
                  n262 = call "Ke2000 Single Reading.vi"("error in (no error)"=w715, "VISA resource name"=w718) -> ("error out"=w713:errorcluster, "VISA resource name out"=w711:refnum<visa-resource-name>, "uA"=w712:string)  [unwired: 5 in, 2 out]
                  n263 = call "Substration.vi"("error in (no error)"=w713, "Input2"=w719, "Input1"=w712) -> ("error out"=w709:errorcluster, "In1 - In2"=w720:string)  [unwired: 7 in]
                }
                n264 = Index Array(array=w648, index=0) -> (element=w650:string)
                n265 = Index Array(array=w648, index=1) -> (element=w647:string)
                n266 = call "Multi Dut Cmd Setting.vi"("error in (no error)"=w646, "Test Seq"="Test Sequences", "Cmin/Act"="Cmin/Act", "WS1050/51"="WS1050/51") -> ("error out"=w662:errorcluster, "Cmd 3"=w656:string[], "Name 3"=w655:string[], "Name Header"=w659:string[], "Cmd 2"=w657:string[], "Name 2"=w660:string[], "Cmd 1"=w658:string[], "Name 1"=w661:string[])
                n267 = local read "SPI Clock Rate (Hz)"() -> (w692:dbl)
              }
              frame #1 {
                n268 = call "WSVCAP SHL Host TL RFFE Configure.vi"("RFFE Slave Address"=w1014, "Clock Rate (Hz)"=w1012, "error in"=w1025) -> ("Actual Rate (Hz)"=w1026:dbl, "error out"=w1000:errorcluster)  [unwired: 11 in]
                n269 = local write "AR  Meas(Hz)"(w1026) -> ()
                n270 = Array Size(array=w1015) -> (size(s)=w1029:i32)
                n271 = call "Delay T4.vi"("milliseconds to wait"=u32 10, "error in (no error)"=w1000) -> ("error out"=w1001:errorcluster)  [unwired: 9 in]
                n272 = case shown="2" w997 {
                  tunnel: w1029 -> [w1037 w1067 w1097]
                  tunnel: w1022 -> [w1036 w1066 w1096]
                  tunnel: [w1035 w1065 w1095] -> w1018
                  tunnel: [w1034 w1064 w1094] -> w1017
                  tunnel: w1016 -> [w1033 w1063 w1093]
                  tunnel: w1015 -> [w1032 w1062 w1092]
                  tunnel: [w1031 w1061 w1091] -> w1006
                  tunnel: w1001 -> [w1030 w1060 w1090]
                  frame 0, Default {
                    n273 = for {
                      N: w1037 -> [_]
                      tunnel: w1033 -> [w1055]
                      tunnel: w1036 -> [w1053]
                      tunnel: [w1052] -> w1035
                      tunnel: [w1048] -> w1034 mode=indexing
                      tunnel: w1032 -> [w1050]
                      tunnel: w1030 -> [w1038]
                      tunnel: [w1040] -> w1031
                      i -> [w1047]
                      stop <- w1052 stop-if-true
                      n274 = Index Array(array=w1055, index=w1047) -> (element=w1051:string)
                      n275 = Index Array(array=w1050, index=w1047) -> (element=w1049:string)
                      n276 = local write "STATUS"(w1049) -> ()
                      n277 = call "WSVCAP SHL Host TL RFFE Write - Multiple DUTs - Common Data.vi"("Data Out"=w1051, "error in"=w1038) -> ("error out"=w1042:errorcluster)  [unwired: 13 in]
                      n278 = call "Delay T4.vi"("milliseconds to wait"=u32 10, "error in (no error)"=w1042) -> ("error out"=w1046:errorcluster)  [unwired: 9 in]
                      n279 = call "WS1050 AD7747 READ.vi"("error in"=w1046, "Log (T)"=FALSE, "DUT Mask Mode (All)"=WSVCAP_SHL_I2C_DUT_Mask_Mode_Enum."C1") -> ("error out"=w1044:errorcluster, "AD7747 Values"=w1045:string[][])  [unwired: 7 in]
                      n280 = for {
                        tunnel: w1045 -> [w1058] mode=indexing
                        tunnel: w1044 -> [w1059]
                        tunnel: [w1059] -> w1040
                        tunnel: [w1056] -> w1048 mode=indexing
                        n281 = Index Array(array=w1058, index=1) -> (element=w1056:string)
                      }
                      n282 = Unbundle By Name(w1040) -> ("status"=w1054:bool)
                      n283 = Or(x=w1054, y=w1053) -> (x .or. y?=w1052:bool)
                    }
                  }
                  frame 1 {
                    n284 = for {
                      N: w1067 -> [_]
                      tunnel: w1063 -> [w1085]
                      tunnel: w1066 -> [w1083]
                      tunnel: [w1082] -> w1065
                      tunnel: [w1078] -> w1064 mode=indexing
                      tunnel: w1062 -> [w1080]
                      tunnel: w1060 -> [w1068]
                      tunnel: [w1070] -> w1061
                      i -> [w1077]
                      stop <- w1082 stop-if-true
                      n285 = Index Array(array=w1085, index=w1077) -> (element=w1081:string)
                      n286 = Index Array(array=w1080, index=w1077) -> (element=w1079:string)
                      n287 = local write "STATUS"(w1079) -> ()
                      n288 = call "WSVCAP SHL Host TL RFFE Write - Multiple DUTs - Common Data.vi"("Data Out"=w1081, "error in"=w1068) -> ("error out"=w1072:errorcluster)  [unwired: 13 in]
                      n289 = call "Delay T4.vi"("milliseconds to wait"=u32 10, "error in (no error)"=w1072) -> ("error out"=w1076:errorcluster)  [unwired: 9 in]
                      n290 = call "WS1050 AD7747 READ.vi"("error in"=w1076, "Log (T)"=FALSE, "DUT Mask Mode (All)"=WSVCAP_SHL_I2C_DUT_Mask_Mode_Enum."C2") -> ("error out"=w1074:errorcluster, "AD7747 Values"=w1075:string[][])  [unwired: 7 in]
                      n291 = for {
                        tunnel: w1075 -> [w1088] mode=indexing
                        tunnel: w1074 -> [w1089]
                        tunnel: [w1089] -> w1070
                        tunnel: [w1086] -> w1078 mode=indexing
                        n292 = Index Array(array=w1088, index=3) -> (element=w1086:string)
                      }
                      n293 = Unbundle By Name(w1070) -> ("status"=w1084:bool)
                      n294 = Or(x=w1084, y=w1083) -> (x .or. y?=w1082:bool)
                    }
                  }
                  frame 2 {
                    n295 = for {
                      N: w1097 -> [_]
                      tunnel: w1093 -> [w1115]
                      tunnel: w1096 -> [w1113]
                      tunnel: [w1112] -> w1095
                      tunnel: [w1108] -> w1094 mode=indexing
                      tunnel: w1092 -> [w1110]
                      tunnel: w1090 -> [w1098]
                      tunnel: [w1100] -> w1091
                      i -> [w1107]
                      stop <- w1112 stop-if-true
                      n296 = Index Array(array=w1115, index=w1107) -> (element=w1111:string)
                      n297 = Index Array(array=w1110, index=w1107) -> (element=w1109:string)
                      n298 = local write "STATUS"(w1109) -> ()
                      n299 = call "WSVCAP SHL Host TL RFFE Write - Multiple DUTs - Common Data.vi"("Data Out"=w1111, "error in"=w1098) -> ("error out"=w1102:errorcluster)  [unwired: 13 in]
                      n300 = call "Delay T4.vi"("milliseconds to wait"=u32 10, "error in (no error)"=w1102) -> ("error out"=w1106:errorcluster)  [unwired: 9 in]
                      n301 = call "WS1050 AD7747 READ.vi"("error in"=w1106, "Log (T)"=FALSE, "DUT Mask Mode (All)"=WSVCAP_SHL_I2C_DUT_Mask_Mode_Enum."C3") -> ("error out"=w1104:errorcluster, "AD7747 Values"=w1105:string[][])  [unwired: 7 in]
                      n302 = for {
                        tunnel: w1105 -> [w1118] mode=indexing
                        tunnel: w1104 -> [w1119]
                        tunnel: [w1119] -> w1100
                        tunnel: [w1116] -> w1108 mode=indexing
                        n303 = Index Array(array=w1118, index=5) -> (element=w1116:string)
                      }
                      n304 = Unbundle By Name(w1100) -> ("status"=w1114:bool)
                      n305 = Or(x=w1114, y=w1113) -> (x .or. y?=w1112:bool)
                    }
                  }
                }
                n306 = Transpose 2D Array(2D array=w1017) -> (transposed array=w1005:string[][])
                "40V_1" <- w1005
                "NOM IDD ON (uA)" <- w1020
                "NOM IDD OFF(uA)" <- w1019
              }
              frame #2 {
                n307 = Array Size(array=w1136) -> (size(s)=w1137:i32)
                n308 = case shown="0, 2, Default" w1121 {
                  tunnel: w1137 -> [w1154 w1184]
                  tunnel: w1136 -> [w1153 w1183]
                  tunnel: [w1152 w1182] -> w1135
                  tunnel: w1134 -> [w1151 w1181]
                  tunnel: w1133 -> [w1150 w1180]
                  tunnel: [w1149 w1179] -> w1132
                  tunnel: [w1148 w1178] -> w1128
                  tunnel: w1126 -> [w1147 w1177]
                  frame 0, 2, Default {
                    n309 = for {
                      N: w1154 -> [_]
                      tunnel: w1151 -> [w1172]
                      tunnel: w1150 -> [w1170]
                      tunnel: [w1169] -> w1149
                      tunnel: [w1165] -> w1152 mode=indexing
                      tunnel: w1153 -> [w1167]
                      tunnel: w1147 -> [w1155]
                      tunnel: [w1157] -> w1148
                      i -> [w1164]
                      stop <- w1169 stop-if-true
                      n310 = Index Array(array=w1172, index=w1164) -> (element=w1168:string)
                      n311 = Index Array(array=w1167, index=w1164) -> (element=w1166:string)
                      n312 = call "WSVCAP SHL Host TL RFFE Write - Multiple DUTs - Common Data.vi"("Data Out"=w1168, "error in"=w1155) -> ("error out"=w1159:errorcluster)  [unwired: 13 in]
                      n313 = local write "STATUS"(w1166) -> ()
                      n314 = call "Delay T4.vi"("milliseconds to wait"=u32 10, "error in (no error)"=w1159) -> ("error out"=w1163:errorcluster)  [unwired: 9 in]
                      n315 = call "WS1050 AD7747 READ.vi"("error in"=w1163, "Log (T)"=FALSE, "DUT Mask Mode (All)"=WSVCAP_SHL_I2C_DUT_Mask_Mode_Enum."C2") -> ("error out"=w1161:errorcluster, "AD7747 Values"=w1162:string[][])  [unwired: 7 in]
                      n316 = for {
                        tunnel: w1162 -> [w1175] mode=indexing
                        tunnel: w1161 -> [w1176]
                        tunnel: [w1176] -> w1157
                        tunnel: [w1173] -> w1165 mode=indexing
                        n317 = Index Array(array=w1175, index=3) -> (element=w1173:string)
                      }
                      n318 = Unbundle By Name(w1157) -> ("status"=w1171:bool)
                      n319 = Or(x=w1171, y=w1170) -> (x .or. y?=w1169:bool)
                    }
                  }
                  frame 1 {
                    n320 = for {
                      N: w1184 -> [_]
                      tunnel: w1181 -> [w1202]
                      tunnel: w1180 -> [w1200]
                      tunnel: [w1199] -> w1179
                      tunnel: [w1195] -> w1182 mode=indexing
                      tunnel: w1183 -> [w1197]
                      tunnel: w1177 -> [w1185]
                      tunnel: [w1187] -> w1178
                      i -> [w1194]
                      stop <- w1199 stop-if-true
                      n321 = Index Array(array=w1202, index=w1194) -> (element=w1198:string)
                      n322 = Index Array(array=w1197, index=w1194) -> (element=w1196:string)
                      n323 = call "WSVCAP SHL Host TL RFFE Write - Multiple DUTs - Common Data.vi"("Data Out"=w1198, "error in"=w1185) -> ("error out"=w1189:errorcluster)  [unwired: 13 in]
                      n324 = local write "STATUS"(w1196) -> ()
                      n325 = call "Delay T4.vi"("milliseconds to wait"=u32 10, "error in (no error)"=w1189) -> ("error out"=w1193:errorcluster)  [unwired: 9 in]
                      n326 = call "WS1050 AD7747 READ.vi"("error in"=w1193, "Log (T)"=FALSE, "DUT Mask Mode (All)"=WSVCAP_SHL_I2C_DUT_Mask_Mode_Enum."C1") -> ("error out"=w1191:errorcluster, "AD7747 Values"=w1192:string[][])  [unwired: 7 in]
                      n327 = for {
                        tunnel: w1192 -> [w1205] mode=indexing
                        tunnel: w1191 -> [w1206]
                        tunnel: [w1206] -> w1187
                        tunnel: [w1203] -> w1195 mode=indexing
                        n328 = Index Array(array=w1205, index=1) -> (element=w1203:string)
                      }
                      n329 = Unbundle By Name(w1187) -> ("status"=w1201:bool)
                      n330 = Or(x=w1201, y=w1200) -> (x .or. y?=w1199:bool)
                    }
                  }
                }
                n331 = Transpose 2D Array(2D array=w1135) -> (transposed array=w1127:string[][])
                "40V_2" <- w1127
              }
              frame #3 {
                n332 = case shown="True" w1209 {
                  tunnel: w1222 -> [_ w1245]
                  tunnel: w1221 -> [_ w1244]
                  tunnel: w1220 -> [w1237 w1239]
                  tunnel: [w1237 w1243] -> w1219
                  tunnel: [string[][] [] w1242] -> w1215
                  tunnel: w1214 -> [w1235 w1241]
                  tunnel: [w1235 w1240] -> w1213
                  tunnel: w1208 -> [_ w1238]
                  frame False {
                  }
                  frame True {
                    n333 = Array Size(array=w1245) -> (size(s)=w1246:i32)
                    n334 = case shown="2" w1238 {
                      tunnel: w1246 -> [w1255 w1286]
                      tunnel: w1245 -> [w1254 w1285]
                      tunnel: w1244 -> [w1253 w1284]
                      tunnel: [w1252 w1283] -> w1243
                      tunnel: [w1250 w1281] -> w1242
                      tunnel: w1241 -> [w1249 w1280]
                      tunnel: [w1248 w1279] -> w1240
                      tunnel: w1239 -> [w1247 w1278]
                      frame 0, 1, Default {
                        n335 = for {
                          N: w1255 -> [_]
                          tunnel: w1253 -> [w1273]
                          tunnel: w1247 -> [w1271]
                          tunnel: [w1270] -> w1252
                          tunnel: [w1266] -> w1251 mode=indexing
                          tunnel: w1254 -> [w1268]
                          tunnel: w1249 -> [w1256]
                          tunnel: [w1258] -> w1248
                          i -> [w1265]
                          stop <- w1270 stop-if-true
                          n336 = Index Array(array=w1273, index=w1265) -> (element=w1269:string)
                          n337 = Index Array(array=w1268, index=w1265) -> (element=w1267:string)
                          n338 = local write "STATUS"(w1267) -> ()
                          n339 = call "WSVCAP SHL Host TL RFFE Write - Multiple DUTs - Common Data.vi"("Data Out"=w1269, "error in"=w1256) -> ("error out"=w1260:errorcluster)  [unwired: 13 in]
                          n340 = call "Delay T4.vi"("milliseconds to wait"=u32 10, "error in (no error)"=w1260) -> ("error out"=w1264:errorcluster)  [unwired: 9 in]
                          n341 = call "WS1050 AD7747 READ.vi"("error in"=w1264, "Log (T)"=FALSE, "DUT Mask Mode (All)"=WSVCAP_SHL_I2C_DUT_Mask_Mode_Enum."C3") -> ("error out"=w1262:errorcluster, "AD7747 Values"=w1263:string[][])  [unwired: 7 in]
                          n342 = for {
                            tunnel: w1263 -> [w1276] mode=indexing
                            tunnel: w1262 -> [w1277]
                            tunnel: [w1277] -> w1258
                            tunnel: [w1274] -> w1266 mode=indexing
                            n343 = Index Array(array=w1276, index=5) -> (element=w1274:string)
                          }
                          n344 = Unbundle By Name(w1258) -> ("status"=w1272:bool)
                          n345 = Or(x=w1272, y=w1271) -> (x .or. y?=w1270:bool)
                        }
                        n346 = Transpose 2D Array(2D array=w1251) -> (transposed array=w1250:string[][])
                      }
                      frame 2 {
                        n347 = for {
                          N: w1286 -> [_]
                          tunnel: w1284 -> [w1304]
                          tunnel: w1278 -> [w1302]
                          tunnel: [w1301] -> w1283
                          tunnel: [w1297] -> w1282 mode=indexing
                          tunnel: w1285 -> [w1299]
                          tunnel: w1280 -> [w1287]
                          tunnel: [w1289] -> w1279
                          i -> [w1296]
                          stop <- w1301 stop-if-true
                          n348 = Index Array(array=w1304, index=w1296) -> (element=w1300:string)
                          n349 = Index Array(array=w1299, index=w1296) -> (element=w1298:string)
                          n350 = local write "STATUS"(w1298) -> ()
                          n351 = call "WSVCAP SHL Host TL RFFE Write - Multiple DUTs - Common Data.vi"("Data Out"=w1300, "error in"=w1287) -> ("error out"=w1291:errorcluster)  [unwired: 13 in]
                          n352 = call "Delay T4.vi"("milliseconds to wait"=u32 10, "error in (no error)"=w1291) -> ("error out"=w1295:errorcluster)  [unwired: 9 in]
                          n353 = call "WS1050 AD7747 READ.vi"("error in"=w1295, "Log (T)"=FALSE, "DUT Mask Mode (All)"=WSVCAP_SHL_I2C_DUT_Mask_Mode_Enum."C1") -> ("error out"=w1293:errorcluster, "AD7747 Values"=w1294:string[][])  [unwired: 7 in]
                          n354 = for {
                            tunnel: w1294 -> [w1307] mode=indexing
                            tunnel: w1293 -> [w1308]
                            tunnel: [w1308] -> w1289
                            tunnel: [w1305] -> w1297 mode=indexing
                            n355 = Index Array(array=w1307, index=1) -> (element=w1305:string)
                          }
                          n356 = Unbundle By Name(w1289) -> ("status"=w1303:bool)
                          n357 = Or(x=w1303, y=w1302) -> (x .or. y?=w1301:bool)
                        }
                        n358 = Transpose 2D Array(2D array=w1282) -> (transposed array=w1281:string[][])
                      }
                    }
                  }
                }
                "40V_3" <- w1215
                n359 = case shown="False" w1209 {
                  tunnel: ["DeltaC Target(pF)_51" "DeltaC Target(pF)_50"] -> w1218
                  frame False {
                  }
                  frame True {
                  }
                }
              }
              frame #4 {
                # "VPI Testing @ 35V"
                n360 = call "WS1050 Delta C Calculation.vi"("WS1050/51"=w1312, "error in (no error)"=w1347, "DCap Target(pF)"=w1346, "Input"=w1349) -> ("error out"=w1344:errorcluster, "Total Bank Delta C(pF)"=w1337:string[], "% Bank DeltaC"=w1341:string[])  [unwired: 3 in, 2 out]
                n361 = call "WS1050 Delta C Calculation.vi"("WS1050/51"=w1311, "error in (no error)"=w1347, "DCap Target(pF)"=w1346, "Input"=w1348) -> ("error out"=w1345:errorcluster, "Total Bank Delta C(pF)"=w1336:string[], "% Bank DeltaC"=w1339:string[])  [unwired: 3 in, 2 out]
                n362 = call "WS1050 Delta C Calculation.vi"("WS1050/51"=w1310, "error in (no error)"=w1347, "DCap Target(pF)"=w1346, "Input"=w1340) -> ("error out"=w1343:errorcluster, "Total Bank Delta C(pF)"=w1335:string[], "% Bank DeltaC"=w1338:string[])  [unwired: 3 in, 2 out]
                n363 = Merge Errors(w1344, w1345, w1343) -> (w1342:errorcluster)
                n364 = case shown="1, Default" w1350 {
                  tunnel: w1342 -> [w1378 w1386]
                  tunnel: [w1378 w1386] -> w1314
                  tunnel: w1341 -> [w1374 w1382]
                  tunnel: w1339 -> [w1373 w1381]
                  tunnel: w1338 -> [w1372 w1380]
                  tunnel: w1337 -> [w1377 w1385]
                  tunnel: [w1377 w1385] -> w1334
                  tunnel: w1336 -> [w1376 w1384]
                  tunnel: [w1376 w1384] -> w1333
                  tunnel: w1335 -> [w1375 w1383]
                  tunnel: [w1375 w1383] -> w1332
                  frame 0 {
                    n365 = Build Array(w1374, w1373, w1372) -> (→"% Delta C_T0":string[][])
                  }
                  frame 1, Default {
                    n366 = Build Array(w1382, w1381, w1380) -> (→"% Delta C":string[][])
                  }
                }
                "Total Delta 1(pF)" <- w1334
                "Total Delta 2(pF)" <- w1333
                "Total Delta 3(pF)" <- w1332
                n367 = call "Multi Dut Cmd VPI Setting.vi"("error in (no error)"=w1314, "Cmin/Act"=w1309, "WS1050/51"=w1312) -> ("error out"=w1313:errorcluster, "Cmd VPI C3"=w1315:string[], "VPI_C3"=w1319:string[], "Name Header VPI"=w1318:string[], "Cmd VPI C2"=w1316:string[], "VPI_C2"=w1320:string[], "Cmd VPI C1"=w1317:string[], "VPI_C1"=w1321:string[])  [unwired: 1 in]
                n368 = case shown="True" w1324 {
                  tunnel: w1364 -> [w1392 w1422]
                  tunnel: [w1391 w1403] -> w1328
                  tunnel: [w1389 w1424] -> w1363
                  tunnel: [w1389 w1410] -> w1362
                  tunnel: [w1392 w1408] -> w1360
                  tunnel: w1357 -> [w1394 w1423]
                  tunnel: [w1394 w1423] -> w1356
                  tunnel: w1317 -> [_ w1421]
                  tunnel: w1316 -> [_ w1415]
                  tunnel: w1315 -> [_ w1411]
                  tunnel: [w1389 w1420] -> w1353
                  tunnel: w1321 -> [w1387 w1418]
                  tunnel: w1320 -> [_ w1416]
                  tunnel: w1319 -> [_ w1412]
                  tunnel: ["NA" ("string") w1407] -> w1330
                  tunnel: w1313 -> [w1391 w1399]
                  tunnel: w1312 -> [_ w1398]
                  frame False {
                    n369 = Array Size(array=w1387) -> (size(s)=w1388:i32)
                    n370 = for {
                      N: w1388 -> [_]
                      tunnel: [w1395] -> w1390 mode=indexing
                      n371 = for {
                        N: 16 -> [_]
                        tunnel: ["na"] -> w1395 mode=indexing
                      }
                    }
                    n372 = Transpose 2D Array(2D array=w1390) -> (transposed array=w1389:string[][])
                    n373 = local write "VPI C1"(w1389) -> ()
                    n374 = local write "VPI C2"(w1389) -> ()
                    n375 = local write "VPI C3"(w1389) -> ()
                  }
                  frame True {
                    # "Set CP to 35V"
                    n376 = flat-sequence {
                      tunnel: [w1484] -> w1404
                      tunnel: w1399 -> [w1482]
                      tunnel: [w1489] -> w1407
                      tunnel: w1404 -> [w1488]
                      tunnel: [w1487] -> w1402
                      frame #0 {
                        n377 = call "WSVCAP SHL Host TL RFFE Write - Multiple DUTs - Common Data.vi"("Data Out"="074820", "error in"=w1482) -> ("error out"=w1485:errorcluster)  [unwired: 13 in]
                        n378 = call "Delay T4.vi"("milliseconds to wait"=u32 10, "error in (no error)"=w1485) -> ("error out"=w1484:errorcluster)  [unwired: 9 in]
                      }
                      frame #1 {
                        n379 = case shown="4" "CP VPI" {
                          selector: "CP VPI" -> [w1497 w1502 w1507 w1512 w1516]
                          tunnel: string[] ["07476F", "074776", "074765", "074769", "07477B"] -> [w1498 w1503 w1508 w1513 w1518]
                          tunnel: [w1496 w1501 w1506 w1511 w1517] -> w1492
                          tunnel: [w1494 w1499 w1504 w1509 w1514] -> w1491
                          tunnel: ["35" ("string") "27.5" ("string") "30.5" ("string") "44.0" ("string") "40.25" ("string")] -> w1489
                          tunnel: w1488 -> [w1494 w1499 w1504 w1509 w1514]
                          frame 0, Default {
                            n380 = Index Array(array=w1498, index=w1497) -> (element=w1496:string)
                          }
                          frame 2 {
                            n381 = Index Array(array=w1503, index=w1502) -> (element=w1501:string)
                          }
                          frame 3 {
                            n382 = Index Array(array=w1508, index=w1507) -> (element=w1506:string)
                          }
                          frame 4 {
                            n383 = Index Array(array=w1513, index=w1512) -> (element=w1511:string)
                          }
                          frame 1 {
                            n384 = Index Array(array=w1518, index=w1516) -> (element=w1517:string)
                          }
                        }
                        n385 = call "WSVCAP SHL Host TL RFFE Write - Multiple DUTs - Common Data.vi"("Data Out"=w1492, "error in"=w1491) -> ("error out"=w1487:errorcluster)  [unwired: 13 in]
                      }
                    }
                    n386 = Array Size(array=w1418) -> (size(s)=w1425:i32)
                    n387 = call "Delay T4.vi"("milliseconds to wait"=u32 50, "error in (no error)"=w1402) -> ("error out"=w1401:errorcluster)  [unwired: 9 in]
                    n388 = for {
                      N: w1425 -> [_]
                      tunnel: w1421 -> [w1536]
                      tunnel: w1422 -> [w1534]
                      tunnel: [w1533] -> w1414
                      tunnel: [w1531] -> w1419 mode=indexing
                      tunnel: w1418 -> [w1530]
                      tunnel: w1401 -> [w1519]
                      tunnel: [w1521] -> w1406
                      i -> [w1529]
                      stop <- w1533 stop-if-true
                      n389 = Index Array(array=w1536, index=w1529) -> (element=w1532:string)
                      n390 = Index Array(array=w1530, index=w1529) -> (element=w1528:string)
                      n391 = call "WSVCAP SHL Host TL RFFE Write - Multiple DUTs - Common Data.vi"("Data Out"=w1532, "error in"=w1519) -> ("error out"=w1527:errorcluster)  [unwired: 13 in]
                      n392 = local write "STATUS"(w1528) -> ()
                      n393 = call "Delay T4.vi"("milliseconds to wait"=u32 10, "error in (no error)"=w1527) -> ("error out"=w1523:errorcluster)  [unwired: 9 in]
                      n394 = call "WS1050 AD7747 READ.vi"("error in"=w1523, "Log (T)"=FALSE, "DUT Mask Mode (All)"=WSVCAP_SHL_I2C_DUT_Mask_Mode_Enum."C1") -> ("error out"=w1525:errorcluster, "AD7747 Values"=w1524:string[][])  [unwired: 7 in]
                      n395 = for {
                        tunnel: [w1539] -> w1531 mode=indexing
                        tunnel: w1525 -> [w1538]
                        tunnel: [w1538] -> w1521
                        tunnel: w1524 -> [w1537] mode=indexing
                        n396 = Index Array(array=w1537, index=1) -> (element=w1539:string)
                      }
                      n397 = Unbundle By Name(w1521) -> ("status"=w1535:bool)
                      n398 = Or(x=w1535, y=w1534) -> (x .or. y?=w1533:bool)
                    }
                    n399 = Transpose 2D Array(2D array=w1419) -> (transposed array=w1424:string[][])
                    "VPI C1" <- w1424
                    n400 = Array Size(array=w1416) -> (size(s)=w1417:i32)
                    n401 = for {
                      N: w1417 -> [_]
                      tunnel: w1415 -> [w1477]
                      tunnel: w1414 -> [w1475]
                      tunnel: [w1474] -> w1409
                      tunnel: [w1472] -> w1413 mode=indexing
                      tunnel: w1416 -> [w1471]
                      tunnel: w1406 -> [w1460]
                      tunnel: [w1462] -> w1405
                      i -> [w1470]
                      stop <- w1474 stop-if-true
                      n402 = Index Array(array=w1477, index=w1470) -> (element=w1473:string)
                      n403 = Index Array(array=w1471, index=w1470) -> (element=w1469:string)
                      n404 = call "WSVCAP SHL Host TL RFFE Write - Multiple DUTs - Common Data.vi"("Data Out"=w1473, "error in"=w1460) -> ("error out"=w1468:errorcluster)  [unwired: 13 in]
                      n405 = local write "STATUS"(w1469) -> ()
                      n406 = call "Delay T4.vi"("milliseconds to wait"=u32 10, "error in (no error)"=w1468) -> ("error out"=w1464:errorcluster)  [unwired: 9 in]
                      n407 = call "WS1050 AD7747 READ.vi"("error in"=w1464, "Log (T)"=FALSE, "DUT Mask Mode (All)"=WSVCAP_SHL_I2C_DUT_Mask_Mode_Enum."C2") -> ("error out"=w1466:errorcluster, "AD7747 Values"=w1465:string[][])  [unwired: 7 in]
                      n408 = for {
                        tunnel: [w1480] -> w1472 mode=indexing
                        tunnel: w1466 -> [w1479]
                        tunnel: [w1479] -> w1462
                        tunnel: w1465 -> [w1478] mode=indexing
                        n409 = Index Array(array=w1478, index=3) -> (element=w1480:string)
                      }
                      n410 = Unbundle By Name(w1462) -> ("status"=w1476:bool)
                      n411 = Or(x=w1476, y=w1475) -> (x .or. y?=w1474:bool)
                    }
                    n412 = Transpose 2D Array(2D array=w1413) -> (transposed array=w1420:string[][])
                    "VPI C2" <- w1420
                    n413 = case shown="True" w1398 {
                      tunnel: w1412 -> [_ w1436]
                      tunnel: w1411 -> [_ w1435]
                      tunnel: [string[][] [] w1433] -> w1410
                      tunnel: w1409 -> [w1428 w1432]
                      tunnel: [w1428 w1431] -> w1408
                      tunnel: w1405 -> [w1427 w1430]
                      tunnel: [w1427 w1429] -> w1403
                      frame False {
                      }
                      frame True {
                        n414 = Array Size(array=w1436) -> (size(s)=w1437:i32)
                        n415 = for {
                          N: w1437 -> [_]
                          tunnel: w1435 -> [w1455]
                          tunnel: w1432 -> [w1453]
                          tunnel: [w1452] -> w1431
                          tunnel: [w1450] -> w1434 mode=indexing
                          tunnel: w1436 -> [w1449]
                          tunnel: w1430 -> [w1438]
                          tunnel: [w1440] -> w1429
                          i -> [w1448]
                          stop <- w1452 stop-if-true
                          n416 = Index Array(array=w1455, index=w1448) -> (element=w1451:string)
                          n417 = Index Array(array=w1449, index=w1448) -> (element=w1447:string)
                          n418 = call "WSVCAP SHL Host TL RFFE Write - Multiple DUTs - Common Data.vi"("Data Out"=w1451, "error in"=w1438) -> ("error out"=w1446:errorcluster)  [unwired: 13 in]
                          n419 = local write "STATUS"(w1447) -> ()
                          n420 = call "Delay T4.vi"("milliseconds to wait"=u32 10, "error in (no error)"=w1446) -> ("error out"=w1442:errorcluster)  [unwired: 9 in]
                          n421 = call "WS1050 AD7747 READ.vi"("error in"=w1442, "Log (T)"=FALSE, "DUT Mask Mode (All)"=WSVCAP_SHL_I2C_DUT_Mask_Mode_Enum."C3") -> ("error out"=w1444:errorcluster, "AD7747 Values"=w1443:string[][])  [unwired: 7 in]
                          n422 = for {
                            tunnel: [w1458] -> w1450 mode=indexing
                            tunnel: w1444 -> [w1457]
                            tunnel: [w1457] -> w1440
                            tunnel: w1443 -> [w1456] mode=indexing
                            n423 = Index Array(array=w1456, index=5) -> (element=w1458:string)
                          }
                          n424 = Unbundle By Name(w1440) -> ("status"=w1454:bool)
                          n425 = Or(x=w1454, y=w1453) -> (x .or. y?=w1452:bool)
                        }
                        n426 = Transpose 2D Array(2D array=w1434) -> (transposed array=w1433:string[][])
                      }
                    }
                    "VPI C3" <- w1410
                  }
                }
                n427 = Insert Into Array(array=w1352, new element=w1318) -> (w1351:string[])  [unwired: 1 in]
                n428 = case shown="False" w1329 {
                  tunnel: w1328 -> [w1365 w1369]
                  tunnel: [w1366 w1368] -> w1327
                  frame False {
                    n429 = call "WSVCAP SHL Host TL RFFE Write - Multiple DUTs - Common Data.vi"("Data Out"="074820", "error in"=w1365) -> ("error out"=w1366:errorcluster)  [unwired: 13 in]
                  }
                  frame True {
                    n430 = call "WSVCAP SHL Host TL RFFE Write - Multiple DUTs - Common Data.vi"("Data Out"="074800", "error in"=w1369) -> ("error out"=w1368:errorcluster)  [unwired: 13 in]
                  }
                }
                n431 = call "Delay T4.vi"("milliseconds to wait"=u32 50, "error in (no error)"=w1327) -> ("error out"=w1326:errorcluster)  [unwired: 9 in]
              }
              frame #5 {
                # "VSA Testing"
                n432 = case shown="True" w1542 {
                  tunnel: w1581 -> [w1596 w1605]
                  tunnel: [w1596 w1604] -> w1555
                  tunnel: [w1595 w1611] -> w1571
                  tunnel: w1572 -> [w1595 w1610]
                  tunnel: [w1592 w1608] -> w1560
                  tunnel: [w1592 w1607] -> w1557
                  tunnel: [w1592 w1606] -> w1554
                  tunnel: [w1593 w1609] -> w1561
                  frame False {
                    n433 = for {
                      tunnel: dbl[] [0.0, 0.0, 0.0] -> [w1600] mode=indexing
                      tunnel: [w1598] -> w1593 mode=indexing
                      tunnel: [w1597] -> w1592 mode=indexing
                      n434 = Number To Fractional String(number=w1600) -> (F-format string=w1599:string)  [unwired: 3 in]
                      n435 = for {
                        N: 16 -> [_]
                        tunnel: w1599 -> [w1603]
                        tunnel: [w1603] -> w1598 mode=indexing
                        tunnel: ["na"] -> w1597 mode=indexing
                      }
                    }
                  }
                  frame True {
                    n436 = for {
                      tunnel: "VSA Voltage(V)" -> [w1635] mode=indexing
                      tunnel: [w1639] -> w1611
                      tunnel: w1610 -> [w1637]
                      tunnel: [w1636] -> w1608 mode=indexing
                      tunnel: [w1623] -> w1607 mode=indexing
                      tunnel: [w1632] -> w1609 mode=indexing
                      tunnel: [w1617] -> w1606 mode=indexing
                      tunnel: w1605 -> [w1616]
                      tunnel: [w1615] -> w1604
                      w1614 = FALSE ("Log (T)")
                      w1631 = u16 0 items=["Voltage", "Current"] ("Source Mode  (0: Voltage)")
                      n437 = call "Ke2400 Configure Output.vi"("Source Mode  (0: Voltage)"=w1631, "error in (no error)"=w1616, "Compliance  Level (0.1)"=0.1, "Output Level (0)"=w1635, "VISA resource name"=w1637) -> ("error out"=w1643:errorcluster, "VISA resource name out"=w1641:refnum<visa-resource-name>)  [unwired: 5 in]
                      n438 = Number To Fractional String(number=w1635) -> (F-format string=w1634:string)  [unwired: 3 in]
                      n439 = call "Ke2400 Enable.vi"("error in (no error)"=w1643, "ON/OFF"=TRUE ("Enable Output (T: Enable)"), "VISA resource name"=w1641) -> ("error out"=w1644:errorcluster, "VISA resource name out"=w1639:refnum<visa-resource-name>)  [unwired: 7 in]
                      n440 = call "Delay T4.vi"("milliseconds to wait"=u32 10, "error in (no error)"=w1644) -> ("error out"=w1630:errorcluster)  [unwired: 9 in]
                      n441 = call "WS1050 AD7747 READ.vi"("error in"=w1630, "Log (T)"=w1614, "DUT Mask Mode (All)"=WSVCAP_SHL_I2C_DUT_Mask_Mode_Enum."C1") -> ("error out"=w1627:errorcluster, "AD7747 Values"=w1629:string[][])  [unwired: 7 in]
                      n442 = for {
                        tunnel: w1629 -> [w1655] mode=indexing
                        tunnel: [w1656] -> w1636 mode=indexing
                        tunnel: w1627 -> [w1654]
                        tunnel: [w1654] -> w1626
                        n443 = Index Array(array=w1655, index=1) -> (element=w1656:string)
                      }
                      n444 = for {
                        N: 16 -> [_]
                        tunnel: w1634 -> [w1653]
                        tunnel: [w1653] -> w1632 mode=indexing
                      }
                      n445 = call "WS1050 AD7747 READ.vi"("error in"=w1626, "Log (T)"=w1614, "DUT Mask Mode (All)"=WSVCAP_SHL_I2C_DUT_Mask_Mode_Enum."C2") -> ("error out"=w1624:errorcluster, "AD7747 Values"=w1622:string[][])  [unwired: 7 in]
                      n446 = for {
                        tunnel: w1622 -> [w1650] mode=indexing
                        tunnel: [w1651] -> w1623 mode=indexing
                        tunnel: w1624 -> [w1649]
                        tunnel: [w1649] -> w1621
                        n447 = Index Array(array=w1650, index=3) -> (element=w1651:string)
                      }
                      n448 = call "WS1050 AD7747 READ.vi"("error in"=w1621, "Log (T)"=w1614, "DUT Mask Mode (All)"=WSVCAP_SHL_I2C_DUT_Mask_Mode_Enum."C3") -> ("error out"=w1619:errorcluster, "AD7747 Values"=w1618:string[][])  [unwired: 7 in]
                      n449 = for {
                        tunnel: w1618 -> [w1646] mode=indexing
                        tunnel: [w1647] -> w1617 mode=indexing
                        tunnel: w1619 -> [w1645]
                        tunnel: [w1645] -> w1615
                        n450 = Index Array(array=w1646, index=5) -> (element=w1647:string)
                      }
                    }
                    n451 = local write "STATUS"("VSA Testing...." ("STATUS")) -> ()
                  }
                }
                n452 = Transpose 2D Array(2D array=w1561) -> (transposed array=w1559:string[][])
                n453 = Transpose 2D Array(2D array=w1560) -> (transposed array=w1558:string[][])
                n454 = Transpose 2D Array(2D array=w1557) -> (transposed array=w1556:string[][])
                n455 = Transpose 2D Array(2D array=w1554) -> (transposed array=w1553:string[][])
                n456 = call "WS1050_VSA_Convert_Data.vi"("VSA_C3"=w1553, "error in (no error)"=w1555, "VSA_C2"=w1556, "VSA_C1"=w1558, "Voltage"=w1559) -> ("error out"=w1552:errorcluster, "VSA_V3"=w1549:string[][], "VSA_V2"=w1550:string[][], "VSA_V1"=w1551:string[][])  [unwired: 3 in]
                "VSA_V1" <- w1551
                "VSA_V2" <- w1550
                "VSA_V3" <- w1549
                n457 = case shown="True" w1542 {
                  tunnel: w1571 -> [w1585 w1591]
                  tunnel: [w1585 w1590] -> w1570
                  tunnel: w1552 -> [w1584 w1589]
                  tunnel: [w1584 w1586] -> w1569
                  frame False {
                  }
                  frame True {
                    w1587 = u16 0 items=["Voltage", "Current"] ("Source Mode  (0: Voltage)")
                    n458 = call "Ke2400 Configure Output.vi"("Source Mode  (0: Voltage)"=w1587, "error in (no error)"=w1589, "Output Level (0)"=0.0, "VISA resource name"=w1591) -> ("error out"=w1586:errorcluster, "VISA resource name out"=w1590:refnum<visa-resource-name>)  [unwired: 6 in]
                  }
                }
                n459 = call "Delay T4.vi"("milliseconds to wait"=u32 50, "error in (no error)"=w1569) -> ("error out"=w1568:errorcluster)  [unwired: 9 in]
              }
              frame #6 {
                # "Handshake Check and EFuse Readback"
                n460 = Or(x=w1667, y=w1677) -> (x .or. y?=w1676:bool)
                n461 = Add(x=w1689, y=w1688) -> (x+y=w1675:u64)
                n462 = case shown="True" w1676 {
                  tunnel: w1702 -> [w1715 _]
                  tunnel: w1701 -> [w1714 w1719]
                  tunnel: [w1713 w1719] -> w1700
                  tunnel: w1699 -> [w1712 _]
                  tunnel: w1698 -> [w1711 _]
                  tunnel: w1697 -> [w1710 _]
                  tunnel: [w1706 w1718] -> w1696
                  tunnel: [w1705 w1718] -> w1691
                  tunnel: w1675 -> [w1704 _]
                  tunnel: w1682 -> [w1703 _]
                  frame False {
                    n463 = call "WS1050_16DUT_Handshake Check R1_Record All Regs Ver1.0.vi"("file path (use dialog)"=w1715, "Reg1_Bit Cntrl"="Reg1_Bit Cntrl", "File Name"=w1703, "SN"=w1710, "Loop"=w1704, "error"=w1714, "Lot #"=w1712, "Wafer #"=w1711) -> ("Pass/Fail"=→"EFuse Readback Status":bool[], "EFuse Read back"=w1705:string[], "Status"=w1706:string[], "error out"=w1713:errorcluster)  [unwired: 6 in, 2 out]
                    n464 = case shown="1, Default" w1704 {
                      tunnel: w1705 -> [w1716 w1717]
                      frame 0 {
                        "EFuse RB T0" <- w1716
                      }
                      frame 1, Default {
                        "Current EFuse Read back" <- w1717
                      }
                    }
                    n465 = local write "STATUS"("Hand Shake & EFuse Readback...." ("STATUS")) -> ()
                  }
                  frame True {
                    w1718 = string[] ["NA", "NA", "NA", "NA", "NA", "NA", "NA", "NA", "NA", "NA", "NA", "NA", "NA", "NA", "NA", "NA"] ("EFuse Read back")
                  }
                }
                n466 = Add(x=w1675, y=w1672) -> (x+y=w1673:u64)
                "TTime Completed" <- w1673
                n467 = Number To Engineering String(4:w1673) -> (0:w1687:string)  [unwired: 3 in]
                n468 = Build Array(w1686, w1684, w1683) -> (w1685:string[])
              }
              frame #7 {
                # "Save Data"
                n469 = Increment(x=w1730) -> (x+1=w1729:i32)
                n470 = local write "STATUS"("Saving Data...." ("STATUS")) -> ()
                n471 = Multiply(x=w1729, y=16) -> (x*y=w1724:i32)
                n472 = Path To String(path=w1734) -> (string=w1733:string)
                n473 = Bundle("Test Program"=w1766, "Comment"=w1765, "Data Out"=w1741, "Data Out"=w1740, "Data Out"=w1739, w1738, "Data Out"=w1737, "Data Out"=w1736, "string"=w1735, "Freq(Hz)"=w1722, "Brd #"=w1721) -> ()  [unwired: 1 in, 1 out]
                n474 = case shown="True" "Debug" {
                  tunnel: w1724 -> [w1773 w1776]
                  tunnel: [w1773 w1774] -> w1723
                  frame False {
                  }
                  frame True {
                    n475 = Multiply(x=w1776, y="No of Rows\nFrom Spread Sheet") -> (x*y=w1774:i32)
                  }
                }
                n476 = call "WS1050_16 DUT SData ver1.2.vi"("TMN DC\\CAP Data Log File Path"=w1734, "Lot#"=w1768, "Total Delta C1(pF)"=w1744, "VSA_V1"=w1753, "Wafer#"=w1764, "File Name"=w1727, "Total Delta C2(pF)"=w1743, "error in"=w1771, "EFuse"=w1758, "Data Output C3"=w1746, "Temperature"=w1750, "VSA_V2"=w1754, "VPI C3"=w1748, "Data Output C1"=w1761, "VPI C2"=w1747, "SN"=w1769, "R/W Status"=w1767, "Cap Header"=w1749, "HD/Cycles Completed"=w1757, "Data Output C2"=w1745, "VSA_V3"=w1752, "Current"=w1760, "VPI C1"=w1759, "Total Delta C3(pF)"=w1742) -> ("error out"=w1770:errorcluster)  [unwired: 3 in]
                n477 = Concatenate Strings(w1733, "\\" ("string"), w1727, "_Multi Socket Data.csv" ("string")) -> (w1732:string)
              }
              frame #8 {
                n478 = case shown="True" "Plot Delta Cmin" {
                  tunnel: w1782 -> [w1797 w1813]
                  tunnel: [w1797 w1809] -> w1781
                  tunnel: w1780 -> [_ w1805]
                  tunnel: w1778 -> [_ w1803]
                  tunnel: w1777 -> [_ w1798]
                  frame False {
                  }
                  frame True {
                    n479 = String To Path(string=w1805) -> (path=w1804:path)
                    n480 = call "Delay T4.vi"("milliseconds to wait"=u32 50, "error in (no error)"=w1813) -> ("error out"=w1812:errorcluster)  [unwired: 9 in]
                    n481 = call "16DUT Plot Subvi Ver1.0.vi"("Plot"="Plot", "No of Rows"=w1803, "error in (no error)"=w1812, "WS1050/51"=w1798, "Bank"=enum16{"C1", "C2", "C3"}."C1", "file path (dialog if empty)"=w1804) -> ("error out"=w1807:errorcluster, "Delta C_Min Plot"=→"Min Plot_1":dbl[][])  [unwired: 4 in]
                    n482 = call "16DUT Plot Subvi Ver1.0.vi"("Plot"="Plot", "No of Rows"=w1803, "error in (no error)"=w1807, "WS1050/51"=w1798, "Bank"=enum16{"C1", "C2", "C3"}."C2", "file path (dialog if empty)"=w1804) -> ("error out"=w1808:errorcluster, "Delta C_Min Plot"=→"Min Plot_2":dbl[][])  [unwired: 4 in]
                    n483 = call "16DUT Plot Subvi Ver1.0.vi"("Plot"="Plot", "No of Rows"=w1803, "error in (no error)"=w1808, "WS1050/51"=w1798, "Bank"=enum16{"C1", "C2", "C3"}."C3", "file path (dialog if empty)"=w1804) -> ("error out"=w1809:errorcluster, "Delta C_Min Plot"=→"Min Plot_3":dbl[][])  [unwired: 4 in]
                  }
                }
                n484 = Get Date/Time In Seconds() -> (seconds since 1Jan1904=w1790:timestamp)
                n485 = Get Date/Time String(seconds (now)=w1790, want seconds? (F)=TRUE) -> (date string=→"date string":string, time string=→"Previous Time":string)  [unwired: 1 in]
                n486 = Greater Or Equal?(x=w1786, y="TTF Completed") -> (x >= y?=w1785:bool)
                n487 = Greater Or Equal?(x=w1787, y="Set HD/Cycle \nto Complete") -> (x >= y?=w1794:bool)
                "No of HD/Cycle\nCompleted" <- w1787
              }
            }
            n488 = Increment(x=w533) -> (x+1=→"Loop \ncompleted":i32)
            n489 = call "Delay T4.vi"("milliseconds to wait"=u32 50, "error in (no error)"=w420) -> ("error out"=w421:errorcluster)  [unwired: 9 in]
            n490 = Compound Arithmetic op=OR(w605, w503, w529) -> (w542:bool)
          }
          "Total Time" <- w361
          n491 = Increment(x=w359) -> (x+1=→"Running Loops":i32)
          n492 = local write "No of HD/Cycle\nCompleted"(u64 0 ("No of HD/Cycle\nCompleted")) -> ()
          n493 = Unbundle By Name(w352) -> ("status"=w365:bool)
          n494 = Compound Arithmetic op=OR(w365, w340, w357) -> (w348:bool)
        }
        n495 = for {
          tunnel: w275 -> [w1824]
          tunnel: w305 -> [w1823]
          tunnel: w306 -> [w1820] mode=indexing
          tunnel: [w1815] -> w273
          tunnel: [w1819] -> w304
          n496 = call "E3631A_Voltage Controller updated.vi"("VISA resource name"=w1823, "Channel Controller"=w1820, "Voltage 1"=0.0, "Voltage 2"=3.3, "error in (no error)"=w1824, "Voltage 3"=-3.3) -> ("VISA resource name out"=w1819:refnum<visa-resource-name>, "error out"=w1816:errorcluster)  [unwired: 8 in]
          n497 = call "Delay T4.vi"("milliseconds to wait"=u32 100, "error in (no error)"=w1816) -> ("error out"=w1815:errorcluster)  [unwired: 9 in]
        }
        n498 = VISA Write(VISA resource name=w295, write buffer="SOUR:FUNC VOLT;VOLT:MODE FIX;RANG 100;LEV 0.0;:SENS:FUNC \"CURR\";CURR:PROT 60E-3;RANG 100E-3;:OUTP ON", error in (no error)=w275) -> (VISA resource name out=w293:refnum<visa-resource-name>, error out=w274:errorcluster)  [unwired: 1 out]
        n499 = Merge Errors(w273, w274) -> (w294:errorcluster)
      }
      frame True {
      }
    }
    n500 = local write "stop During HD/Cycles"(w51) -> ()
    n501 = Unbundle By Name(w62) -> ("status"=w52:bool)
    n502 = Compound Arithmetic op=OR(w52, w51, w71) -> (w80:bool)
    n503 = Wait Until Next ms Multiple(millisecond multiple=u32 100) -> ()  [unwired: 1 out]
    "STATUS" <- "Idle...." ("STATUS")
  }
  "Ke2000 Out" <- w30
  "PS1 Out" <- w29
  n504 = local write "stop During HD/Cycles"(w16) -> ()
  n505 = local write "stop"(w16) -> ()
  n506 = case shown="True" w27 {
    tunnel: [w1841 w1843] -> w14
    tunnel: w22 -> [w1841 w1842]
    frame False {
    }
    frame True {
      n507 = flat-sequence {
        tunnel: w1842 -> [w1846]
        tunnel: [w1845] -> w1843
        frame #0 {
          n508 = local write "Online"(FALSE ("Online")) -> ()
          n509 = call "WSVCAP SHL Host TL Close.vi"("error in"=w1846) -> ("error out"=w1845:errorcluster)  [unwired: 14 in]
        }
      }
    }
  }
  "error out" <- w14
  n510 = VISA Write(VISA resource name=w23, write buffer="SOUR:FUNC VOLT;VOLT:MODE FIX;RANG 100;LEV 0.0;:SENS:FUNC \"CURR\";CURR:PROT 60E-3;RANG 100E-3;:OUTP OFF", error in (no error)=w22) -> (VISA resource name out=→"VISA resource name out":refnum<visa-resource-name>, error out=→"error out 2":errorcluster)  [unwired: 1 out]
